vi "SO2 43i Serial Data Recording & DECADEv4.4.vi"() -> ()   [LabVIEW 2014]
uses:
  <vilib>/Instr/_visa.llb/VISA Set IO Buffer Mask.ctl
  <vilib>/Platform/TimedLoop/XDataNode/timing_clust.ctl
  <vilib>/Platform/TimedLoop/XDataNode/nitl_modes.ctl
  <vilib>/Platform/TimedLoop/XDataNode/wakeup.ctl
  C:/Program Files (x86)/National Instruments/LabVIEW 2014/examples/Data Communication/Network Streams/Simple Network Streams/support/Network Stream Command.ctl
  <vilib>/Utility/error.llb/whitespace.ctl
  <vilib>/Instr/_visa.llb/VISA Configure Serial Port (Instr).vi
  <vilib>/Utility/file.llb/Read From Spreadsheet File (string).vi
  <vilib>/Utility/tcp.llb/UDP Multicast Write-Only Open.vi
  <vilib>/platform/TimedLoop/XDataNode/XDataNode.xnode
  <vilib>/Platform/TimedLoop/XDataNode/XDNodeRunTimeDep.lvlib
  <vilib>/ptbypt/NI_PtbyPt.lvlib
panel:
  out "ASCII_file_out":string
  out "local\ndummy":bool
  out "cal gas cylinder conc":dbl=500.0 format="%.4g"
  out "calcon save to file":bool
  out "ev8 zero interval":i32=600
  out "Auto Zeroing":bool
  out "Simulate MOCCA Conc":dbl
  out "MOCCA window delay time (sec)":i32=30
  out "MOCCA SO2 Limit":i32=800
  out "SO2 Inflight MOCCA Alarm\n(default = OFF)":bool
  out "ev8 user set time":i32=60
  out "Mean Cal Offset":dbl
  out "Mean Cal\n(default = ON)":bool=TRUE
  out "Default file name":string
  out "Stop File Write":bool
  out "error out 4":errorcluster
  out "V6":bool
  out "V8":bool
  out "V9":bool
  out "error out 2":errorcluster
  in  "MFC_2 SLPM set value":dbl
  out "Value Read 2":string
  out "status 2":bool
  out "MFC 2":dbl[](array[numeric])
  in  "VISA resource name 3":refnum<visa-resource-name>="ASRL4::INSTR"
  in  "timeout (10sec) 3":u32=3000
  out "error out 3":errorcluster
  in  "MFC_3 SLPM set value":dbl=2.0
  out "Value Read 3":string
  out "status":bool
  out "MFC 3":dbl[](array[numeric])
  in  "VISA resource name 2":refnum<visa-resource-name>="ASRL5::INSTR"
  in  "timeout (10sec) 2":u32=3000
  out "Data Array UDP":string[](array[string])
  out "Slope":dbl=1.1
  out "Zero":dbl
  out "Simulate TWA Conc":dbl
  out "8hr_TWA_limit":i32=490
  out "10mins_STEL_limit":i32=800
  out "Simulate STEL Conc":dbl
  out "Simulate\nconc":bool
  out "q_size 2":i32
  out "8hr_so2_avg 2":dbl=1.0
  out "10min_so2_avg":dbl=1.0
  out "q_size":i32
  in  "Clear Display\nErrors":bool
  out "Data Processing":bool
  out "Serial Visa Error":errorcluster
  out "SEPTIC TCP Error Out":errorcluster
  out "TCP packet\nSend to SEPTIC":bool
  out "UDP Time Stamp Offset":i32=1
  out "Data Array TCP":string[](array[string])
  out "UDP packet \nstatus":bool
  out "UDP_Out_Error":errorcluster
  out "FISH TCP Error Out":errorcluster
  out "TCP packet\nSend to FISH":bool
  out "TCP Binary Packet":string
  out "Scan from String Error Counter\nfrom process loop":i32
  out "Read Error Counter\nfrom process loop":i32
  in  "milliseconds to wait":u32=330
  in  "ID":string="µ"
  in  "VISA resource name":refnum<visa-resource-name>="ASRL6::INSTR"
  out "Data In Array":string[](array[string])
  out "UDP_ASCII_Out":string
  out "UDP_Pack_num":u32
  out "Flight Number":string
  in  "dummy":string="00"
  out "Data String":string
  out "Internal packet":string[](array[string])
  out "RAW DATA":string
  in  "stop":bool
  out "Time taken history":u32(graph)
  out "Max Acq Time diff":u32
  out "Acq Time":u32
  out "Number of Send & Read Error\nfrom Acquire Loop":i32
  out "Command In":string
  # "SO2_conc"
  # "PMT_Volt"
  # "Lamp_Volt"
  # "Lamp_Intensity_Hz"
  # "Internal_Temp_degC"
  # "Reaction_Chamber_Temp_degC"
  # "Reaction_Chamber_Press_mmHg"
  # "Sample_Flow_litre_per_minute"
  # "Flag"
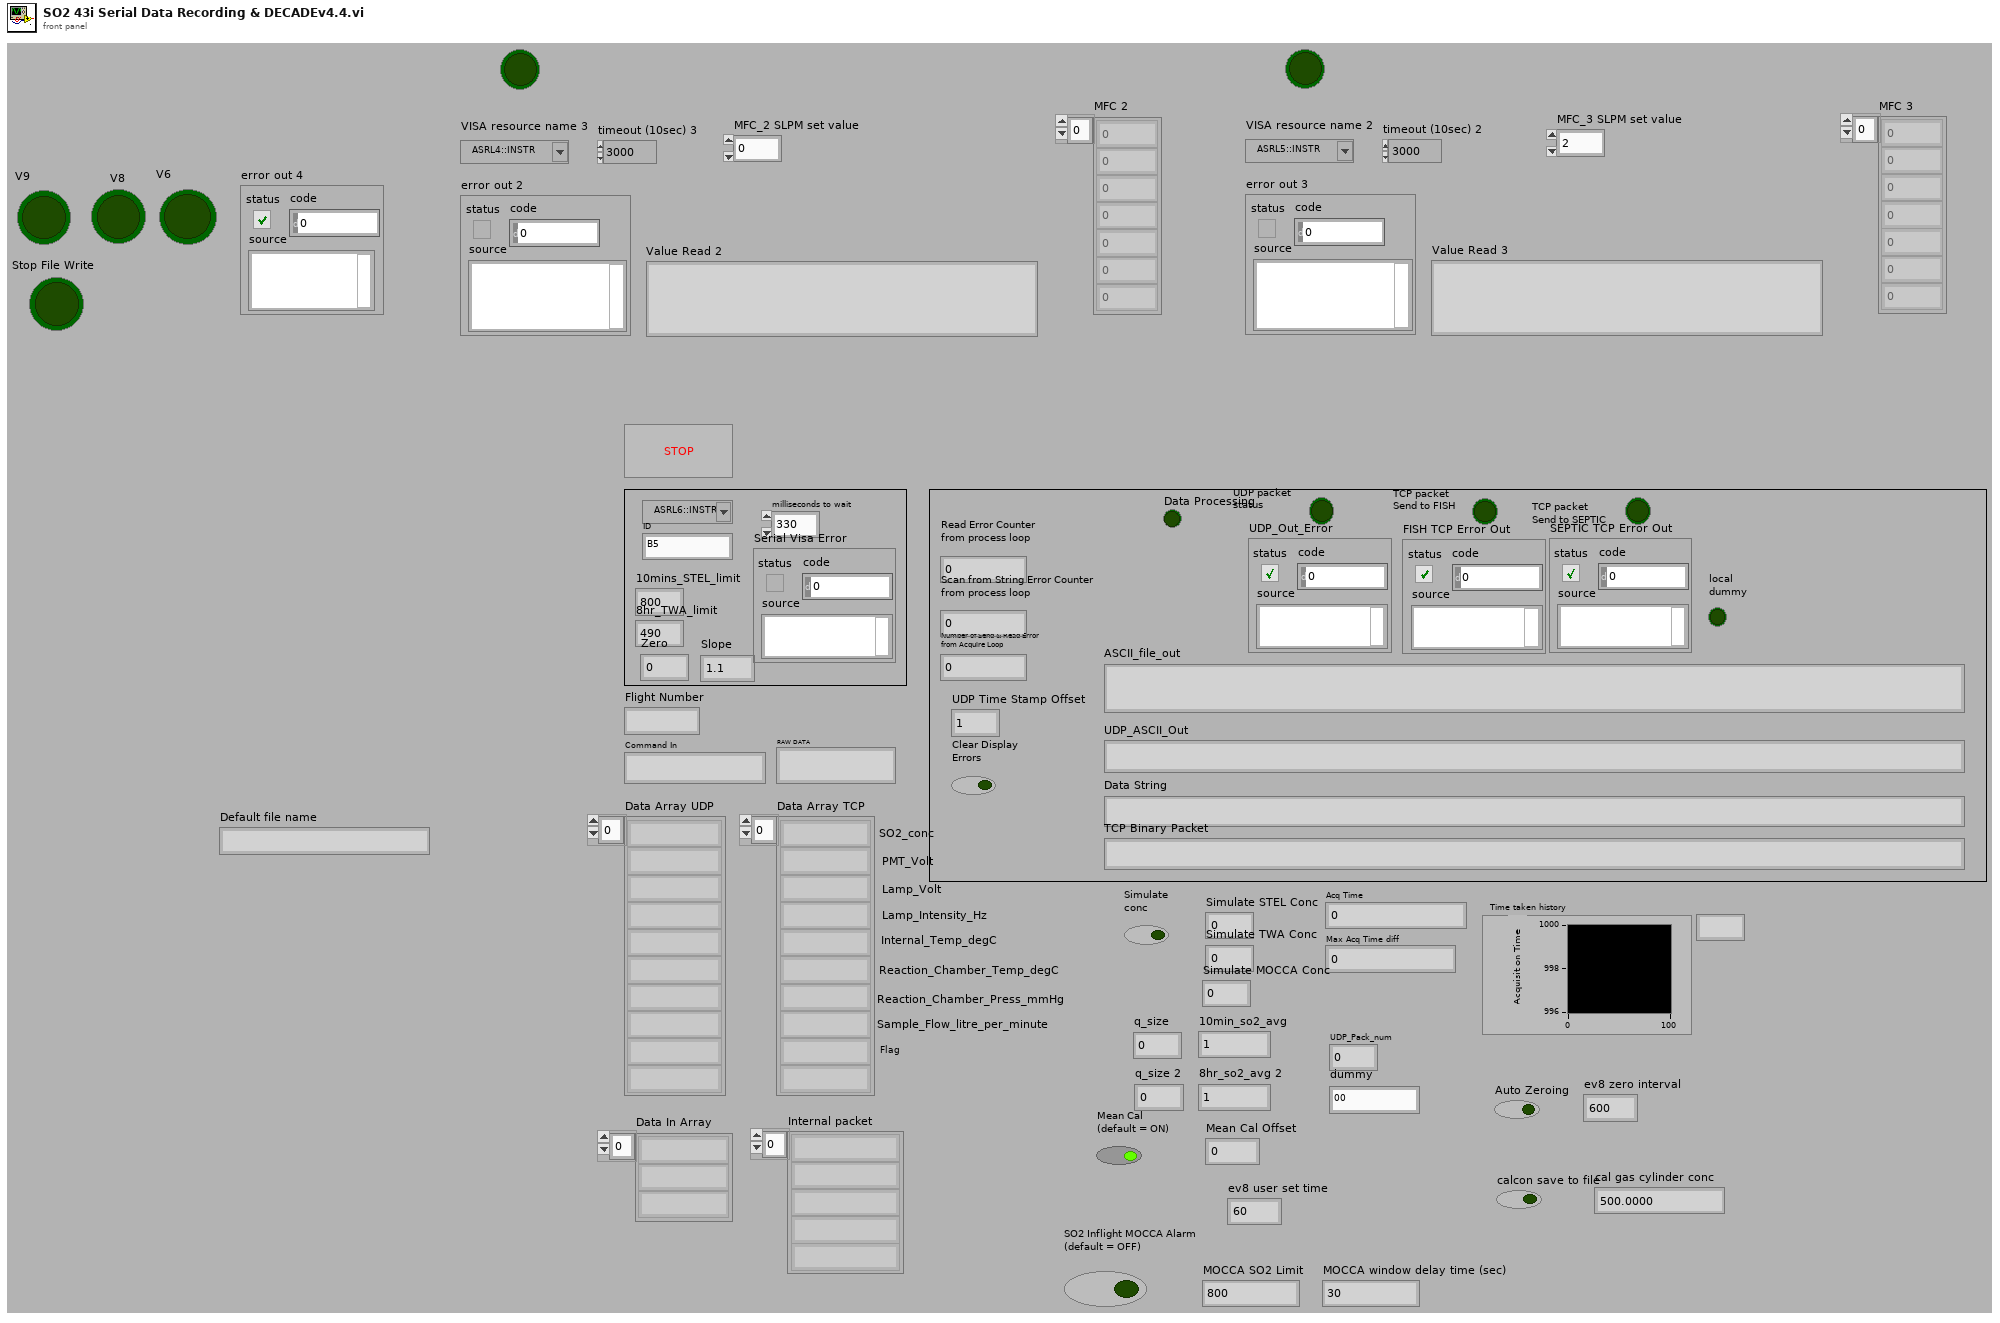
[diagram p1: front panel]
types:
  T1 = typedef "VISA Set IO Buffer Mask.ctl" = u16
  T2 = enum16{"open", "replace", "create", "open or create", "replace or create", "replace or create with confirmation"}
  T3 = typedef "Network Stream Command.ctl" = cluster{"Message":string, "Message Data":variant}
  T4 = typedef "XDNodeRunTimeDep.lvlib/timing_clust.ctl" = cluster{"Expected End [f-1]":u64, "Actual End [f-1]":u64, "Finished Late? [f-1]":bool, "Expected End [i-1]":u64, "Actual End [i-1]":u64, "Finished Late? [i-1]":bool, "Expected Start [i]":u64, "Actual Start [i]":u64, "Expected Start [f]":u64, "Actual Start [f]":u64, "Source Name":string, "Structure Name":string, "Period":i64, "Deadline":i64, "Offset":i64, "Start":i64, "Priority":i32, "Timeout":i32, "Mode":T5, "Wakeup Reason":T6, "Error":errorcluster, "Source Type":string, "Secondary Source Type":string, "Global End Time":u64, "Global Start Time":u64, "Frame Duration":u64, "Iteration Duration":u64, "Assigned CPU":i32, "I/O Scan Engine Mode":u32}
  T5 = typedef "XDNodeRunTimeDep.lvlib/nitl_modes.ctl" = enum32{"No Change", "Process missed periods, maintain original phase", "Discard missed periods, maintain original phase", "Process missed periods, ignore original phase", "Discard missed periods, ignore original phase"}
  T6 = typedef "XDNodeRunTimeDep.lvlib/wakeup.ctl" = enum32{"Normal", "Aborted", "Asynchronous wakeup", "Timing source error", "Timed loop error", "Timeout"}
  T7 = typedef "whitespace.ctl" = u16
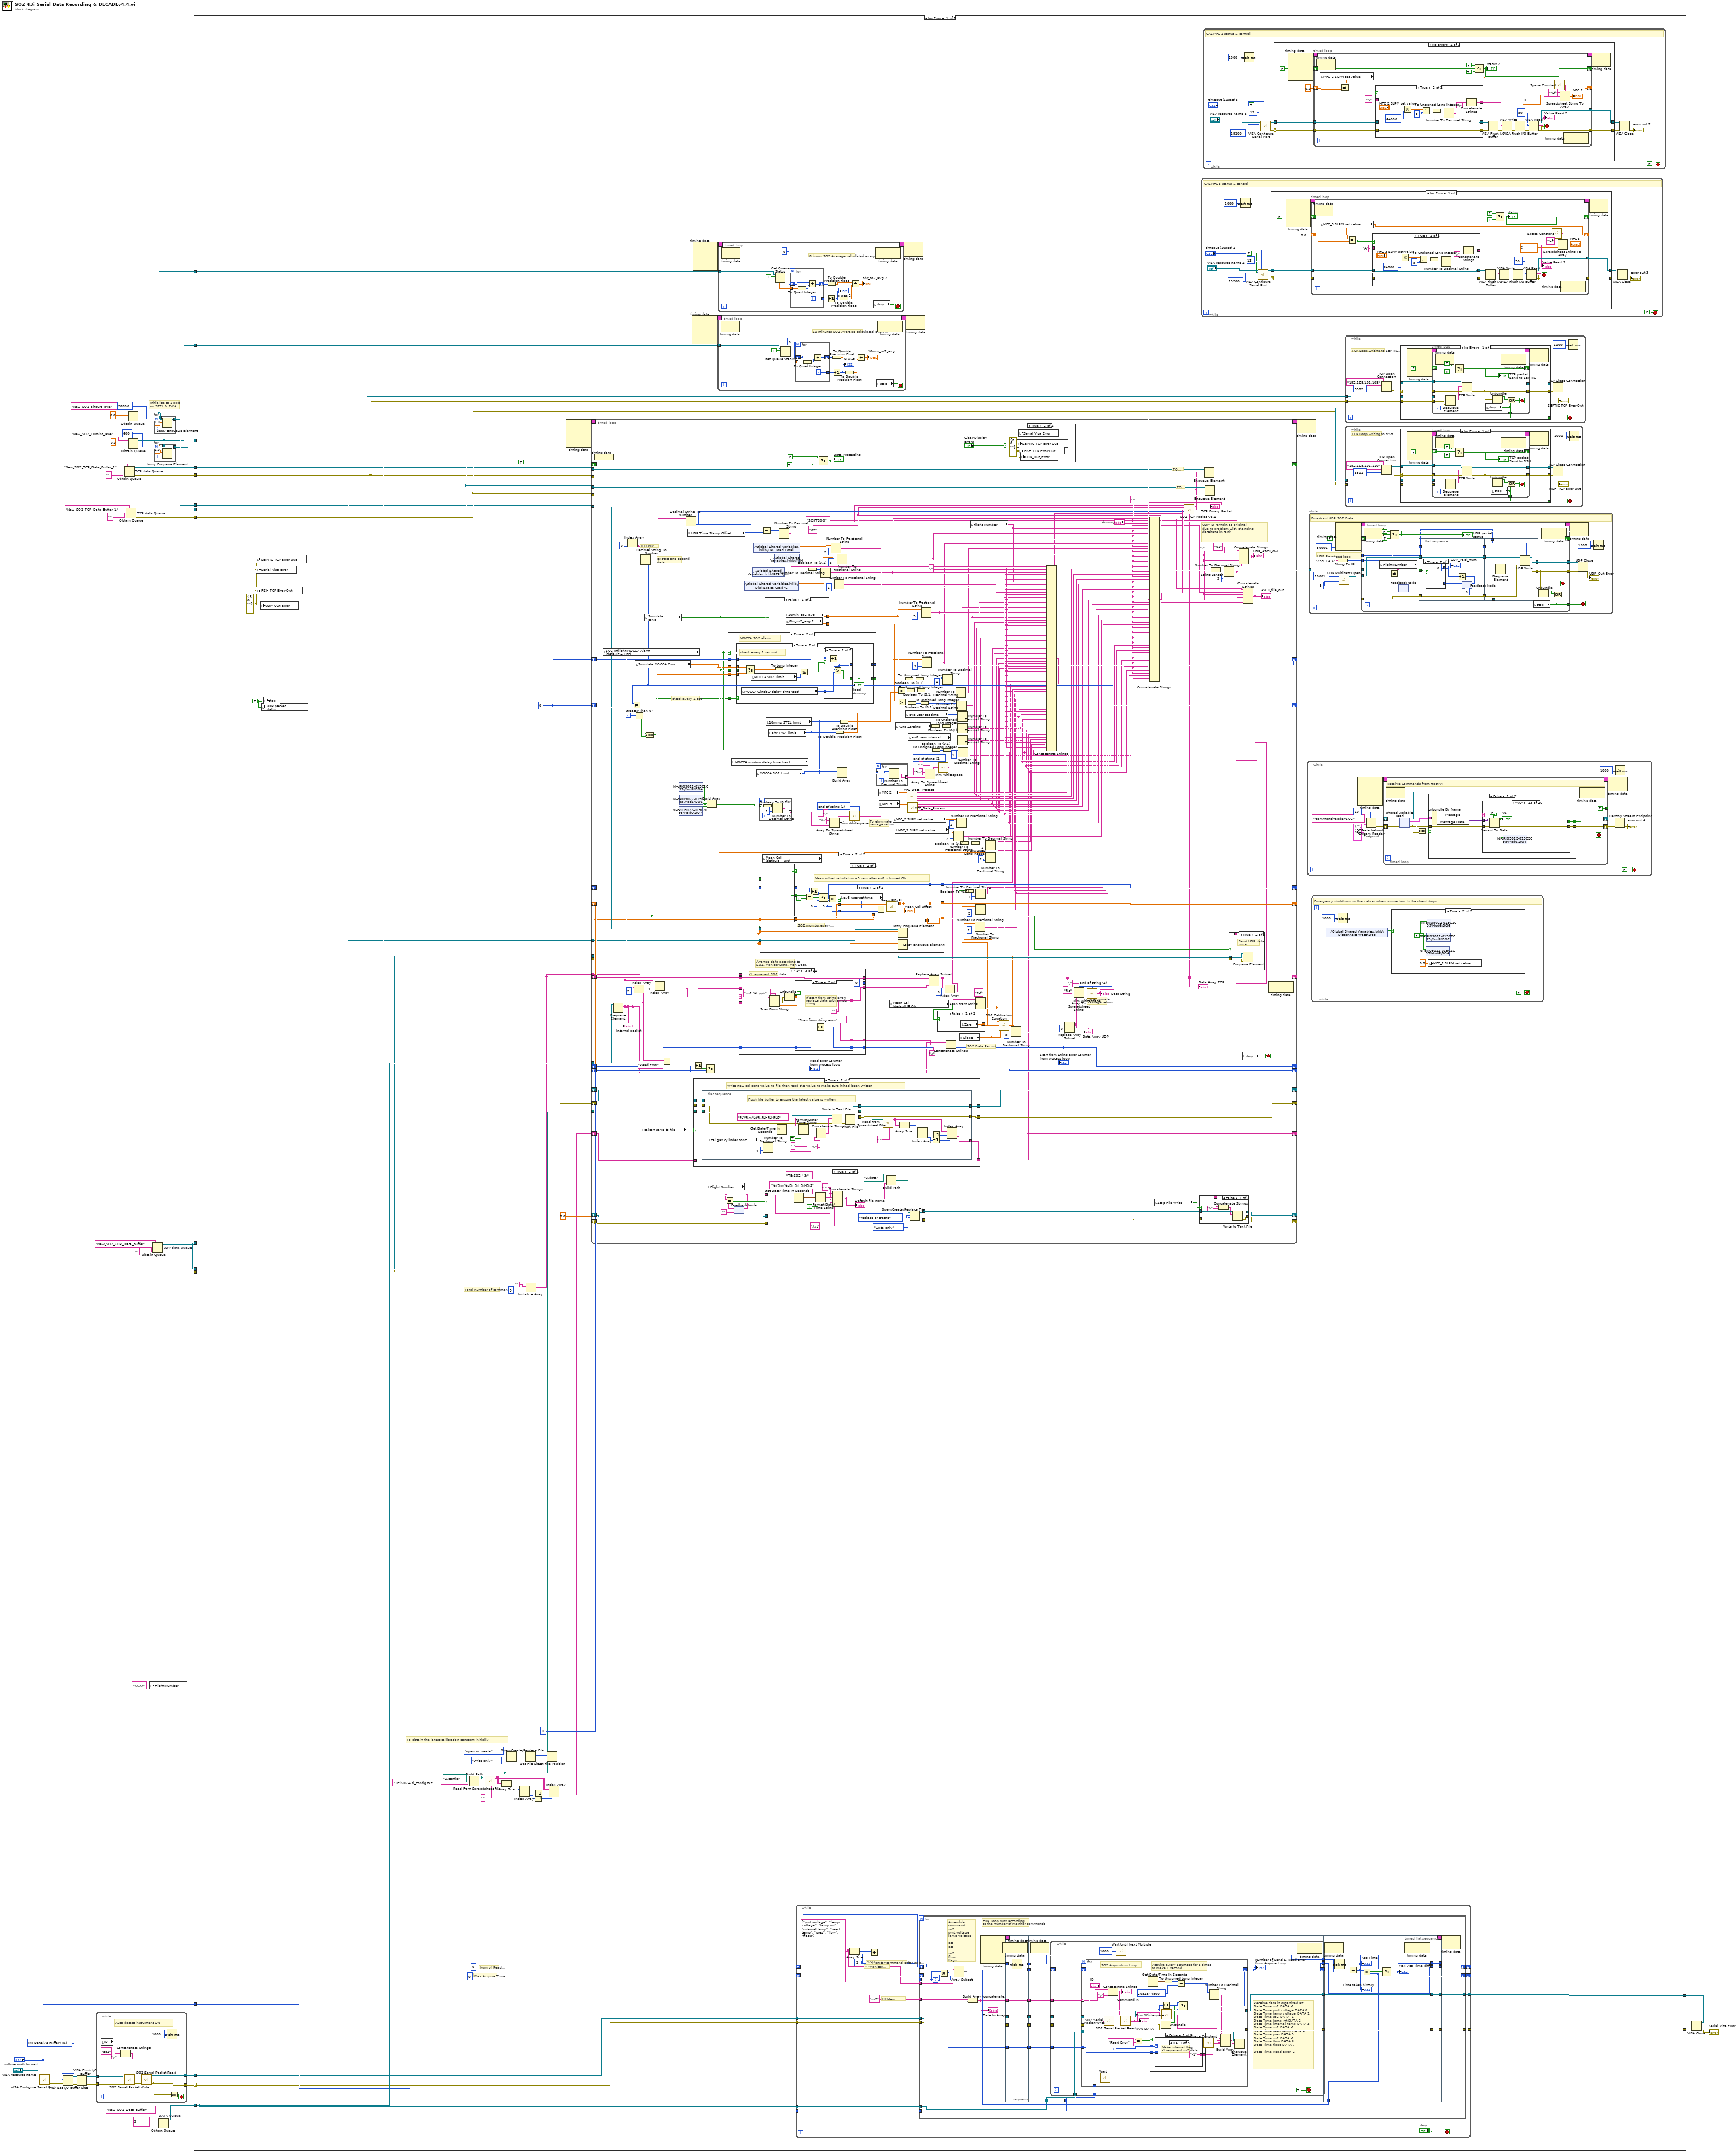
[diagram p0: block diagram]
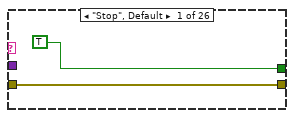
[diagram p3: hidden frame]
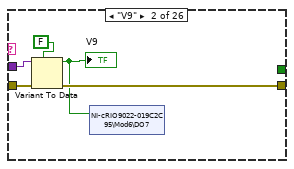
[diagram p4: hidden frame]
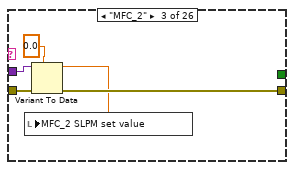
[diagram p5: hidden frame]
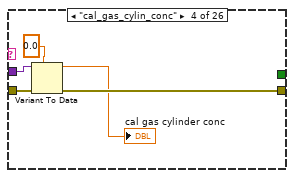
[diagram p6: hidden frame]
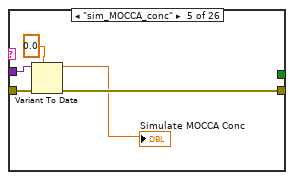
[diagram p7: hidden frame]
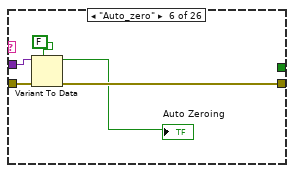
[diagram p8: hidden frame]
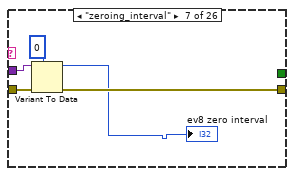
[diagram p9: hidden frame]
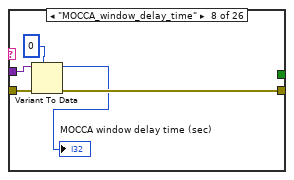
[diagram p10: hidden frame]
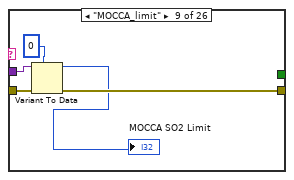
[diagram p11: hidden frame]
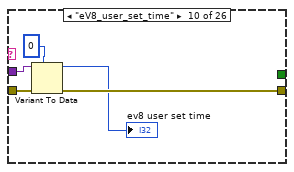
[diagram p12: hidden frame]
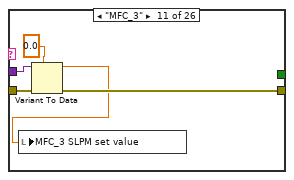
[diagram p13: hidden frame]
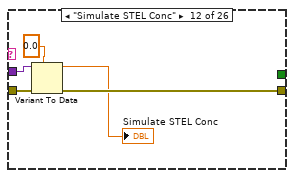
[diagram p14: hidden frame]
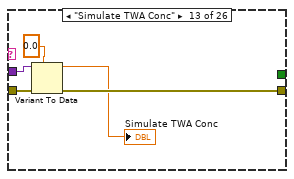
[diagram p15: hidden frame]
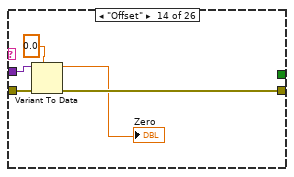
[diagram p16: hidden frame]
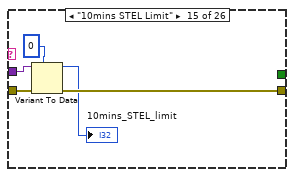
[diagram p17: hidden frame]
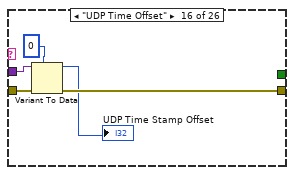
[diagram p18: hidden frame]
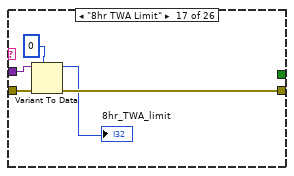
[diagram p19: hidden frame]
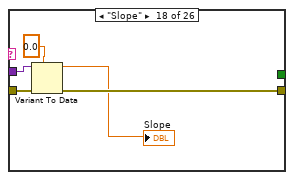
[diagram p20: hidden frame]
diagram:
  w9 = T1 16 items=["I/O Receive Buffer"=16, "I/O Transmit Buffer"=32, "I/O Receive and Transmit Buffer"=48] ("Mask")
  w16 = 28800 ("max queue size (-1, unlimited)")
  w13 = 600 ("max queue size (-1, unlimited)")
  # "Initialise to 1 ppb\non STEL & TWA"
  n1 = call-poly "VISA Configure Serial Port"("VISA resource name"="VISA resource name", "timeout (10sec)"="milliseconds to wait") -> ("VISA resource name out"=w8:refnum<visa-resource-name>, "error out"=w7:errorcluster)  [unwired: 12 in]
  n2 = VISA Set I/O Buffer Size(VISA resource name=w8, mask (16)=w9, error in (no error)=w7) -> (VISA resource name out=w2:refnum<visa-resource-name>, error out=w10:errorcluster)  [unwired: 1 in]
  n3 = VISA Flush I/O Buffer(VISA resource name=w2, error in (no error)=w10) -> (VISA resource name out=w6:refnum<visa-resource-name>, error out=w5:errorcluster)  [unwired: 1 in]
  n4 = while {
    tunnel: w6 -> [w45]
    tunnel: w5 -> [w44]
    tunnel: [w43] -> w4
    tunnel: [w42] -> w3
    stop <- w41 stop-if-true
    # "Auto detect instrument ON"
    n5 = local read "ID"() -> (w46:string)
    n6 = Concatenate Strings(w46, "so2" ("string"), "\r") -> (w49:string)
    n7 = call "SO2 Serial Packet Write.vi"("VISA resource name In"=w45, "Data in"=w49, "error in (no error)"=w44) -> ("VISA resource name Out"=w51:refnum<visa-resource-name>, "error out"=w50:errorcluster)  [unwired: 11 in]
    n8 = call "SO2 Serial Packet Read.vi"("VISA resource In"=w51, "error in"=w50) -> ("VISA resource Out"=w42:refnum<visa-resource-name>, "error out"=w43:errorcluster)  [unwired: 11 in, 1 out]
    n9 = Wait (ms)(milliseconds to wait=u32 1000) -> ()  [unwired: 1 out]
    n10 = Not(x=w43) -> (.not. x?=w41:bool)
  }
  n11 = Obtain Queue "TCP data Queue"(name (unnamed)="New_SO2_TCP_Data_Buffer_2", element data type="") -> (queue out=w23:refnum<queue>, error out=w22:errorcluster)  [unwired: 3 in, 1 out]
  n12 = Obtain Queue "TCP data Queue"(name (unnamed)="New_SO2_TCP_Data_Buffer_1", element data type="") -> (queue out=w31:refnum<queue>, error out=w30:errorcluster)  [unwired: 3 in, 1 out]
  n13 = Obtain Queue(max queue size (-1, unlimited)=w16, name (unnamed)="New_SO2_8hours_ave", element data type=0.0 ("index")) -> (queue out=w15:refnum<queue>)  [unwired: 2 in, 2 out]
  n14 = Obtain Queue(max queue size (-1, unlimited)=w13, name (unnamed)="New_SO2_10mins_ave", element data type=0.0 ("index")) -> (queue out=w12:refnum<queue>)  [unwired: 2 in, 2 out]
  n15 = local write "Flight Number"("XXXX" ("Flight Number")) -> ()
  n16 = Obtain Queue "UDP data Queue"(name (unnamed)="New_SO2_UDP_Data_Buffer", element data type="") -> (queue out=w26:refnum<queue>, error out=w27:errorcluster)  [unwired: 3 in, 1 out]
  n17 = for {
    N: w16 -> [_]
    tunnel: w15 -> [w55]
    tunnel: [w54] -> w14
    n18 = Lossy Enqueue Element(queue=w55, element=1.0) -> (queue out=w54:refnum<queue>)  [unwired: 1 in, 3 out]
  }
  n19 = for {
    N: w13 -> [_]
    tunnel: [w58] -> w11
    tunnel: w12 -> [w56]
    n20 = Lossy Enqueue Element(queue=w56, element=1.0) -> (queue out=w58:refnum<queue>)  [unwired: 1 in, 3 out]
  }
  n21 = Obtain Queue "DATA Queue"(name (unnamed)="New_SO2_Data_Buffer", element data type=string[] []) -> (queue out=w38:refnum<queue>)  [unwired: 3 in, 2 out]
  n22 = case shown="No Error" w4 {
    selector: w4 -> [w81 w1298]
    tunnel: [w112 w1298] -> w35
    tunnel: [w111 w1297] -> w36
    tunnel: w38 -> [w108 _]
    tunnel: w3 -> [w82 w1297]
    tunnel: w31 -> [w100 _]
    tunnel: w30 -> [w99 _]
    tunnel: w26 -> [w98 _]
    tunnel: w27 -> [w97 _]
    tunnel: w26 -> [w96 _]
    tunnel: w23 -> [w95 _]
    tunnel: w22 -> [w94 _]
    tunnel: "milliseconds to wait" -> [w93 _]
    tunnel: w12 -> [w90 _]
    tunnel: w15 -> [w89 _]
    tunnel: w11 -> [w88 _]
    tunnel: w14 -> [w87 _]
    frame No Error {
      w79 = 0
      w91 = errorcluster {"status"=FALSE, "code"=0, "source"=""} ("UDP Error Out")
      w102 = 0
      w101 = FALSE ("stop")
      # "To obtain the latest calibration constant initially"
      # "Max Acquire Time Diff"
      # "Num of Read Error"
      # "Total number of commands"
      n23 = local write "SEPTIC TCP Error Out"(w91) -> ()
      n24 = local write "Serial Visa Error"(w91) -> ()
      n25 = local write "FISH TCP Error Out"(w91) -> ()
      n26 = local write "UDP_Out_Error"(w91) -> ()
      n27 = local write "UDP packet \nstatus"(w101) -> ()
      n28 = local write "stop"(w101) -> ()
      n29 = Build Path(base path=path "u:/config", name or relative path="TEiSO2-43i_config.txt" ("string")) -> (appended path=w61:path)
      n30 = call-poly <vilib>:"Read From Spreadsheet File.vi"("delimiter (\\t)"="," ("delimiter (\\t)"), "file path (dialog if empty)"=w61) -> ("all rows"=w70:string[][])  [unwired: 5 in, 4 out]
      n31 = Array Size(array=w70) -> (size(s)=w71:i32[])
      n32 = Open/Create/Replace File(file path (use dialog)=w61, operation (0:open)=T2."open or create", access (0:read/write)=enum16{"read/write", "read-only", "write-only"}."write-only") -> (refnum out=w63:refnum<file>, error out=w64:errorcluster)  [unwired: 3 in, 1 out]
      n33 = Index Array(array=w71) -> (element #1=w75:i32, element #2=w73:i32)  [unwired: 2 in]
      n34 = Get File Size(file=w63, error in=w64) -> (refnum out=w65:refnum<file>, size (in bytes)=w67:i64, 0:w66:errorcluster)
      n35 = Initialize Array("", 9) -> (w103:string[])
      n36 = Decrement(x=w73) -> (x-1=w72:i32)
      n37 = Decrement(x=w75) -> (x-1=w74:i32)
      n38 = Set File Position(offset (in bytes) (0)=w67, refnum=w65, error in=w66) -> (refnum out=w60:refnum<file>, error out=w59:errorcluster)  [unwired: 1 in]
      n39 = Index Array(array=w70, index (row)=w74, index (col)=w72) -> (element=w69:string)
      n40 = node-c288() -> (w110:T4)  [unwired: 4 in]
      n41 = timed-loop {
        timing: w110 -> [_]
        timing-out: [_] -> w109
        tunnel: w108 -> [w947]
        shift-right: [w745] -> _
        shift-left: w103 -> [w940]
        shift-right: [w931] -> _
        shift-left: w102 -> [w928]
        tunnel: w103 -> [w930]
        shift-right: [w926] -> _
        shift-left: w102 -> [w927]
        tunnel: w100 -> [w924]
        tunnel: w99 -> [w923]
        tunnel: w98 -> [w922]
        tunnel: w97 -> [w921]
        shift-right: [w913] -> _
        shift-left: w79 -> [w916]
        tunnel: w95 -> [w912]
        tunnel: w94 -> [w911]
        shift-right: [w904] -> _
        shift-left: FALSE -> [w907]
        tunnel: w88 -> [w901]
        tunnel: w87 -> [w900]
        shift-right: [w870] -> _
        shift-left: _ -> [w872]
        shift-right: [w869] -> _
        shift-left: _ -> [w871]
        shift-right: [w840] -> _
        shift-left: w79 -> [w842]
        shift-right: [w838] -> _
        shift-left: 0.0 -> [w839]
        shift-right: [w828] -> _
        shift-left: w79 -> [w829]
        tunnel: w61 -> [w805]
        shift-right: [w759] -> _
        shift-left: w69 -> [w804]
        shift-right: [w795] -> _
        shift-left: w60 -> [w796]
        shift-right: [w793] -> _
        shift-left: w59 -> [w794]
        i -> [w914]
        stop <- w945 stop-if-true
        w756 = ","
        (unwired) i16 1 ("width (-)")
        (unwired) T7 2 items=["both", "start of string", "end of string"] ("location (both)")
        w848 = T7 2 items=["both", "start of string", "end of string"] ("location (both)")
        w936 = T7 2 items=["both", "start of string", "end of string"] ("location (both)")
        w798 = ","
        w749 = "02"
        w750 = ","
        w748 = "$CHTSOO"
        # "UDP ID remain as original\ndue to problem with changing\ndatabase in tank"
        # "check every 1 sec"
        # "To eliminate\ncarriage return"
        # "TO SEPTIC"
        # "TO FISH"
        # "Extract one second data\nfor UDP sending"
        # "Arrange data according to\nSO2, Monitor Data, Mon Data,"
        # "To eliminate\ncarriage return"
        # ">>UNIX TIME>>"
        # "SO2 Data Record"
        n42 = node-c288() -> ()  [unwired: 1 in]
        n43 = local read "SO2 Inflight MOCCA Alarm\n(default = OFF)"() -> (w791:bool)
        n44 = Dequeue Element(queue=w947) -> (element=w919:string[])  [unwired: 2 in, 3 out]
        "Internal packet" <- w919
        n45 = Index Array(array=w919, index=0) -> (element=w918:string)
        n46 = Index Array(array=w919, index=2) -> (element=w934:string)
        n47 = Greater Than 0?(x=w914) -> (x > 0?=w917:bool)
        n48 = local read "Simulate MOCCA Conc"() -> (w799:dbl)
        n49 = Decimal String To Number(string=w918) -> (number=w913:i32)  [unwired: 2 in, 1 out]
        n50 = Not Equal?(x=w913, y=w916) -> (x != y?=w915:bool)
        n51 = local read "calcon save to file"() -> (w792:bool)
        n52 = local read "Simulate\nconc"() -> (w801:bool)
        n53 = Compound Arithmetic op=AND(w915, w917) -> (w790:bool)
        n54 = Index Array(array=w919, index=4) -> (element=w903:string)
        n55 = Equal?(x=w934, y="Read Error") -> (x = y?=w932:bool)
        n56 = shared-variable "NI-cRIO9022-019C2C95\\Mod6\\DO7"() -> (w856:bool)  [unwired: 1 in, 1 out]
        n57 = shared-variable "NI-cRIO9022-019C2C95\\Mod6\\DO4"() -> (w857:bool)  [unwired: 1 in, 1 out]
        n58 = shared-variable "NI-cRIO9022-019C2C95\\Mod6\\DO6"() -> (w843:bool)  [unwired: 1 in, 1 out]
        n59 = Decimal String To Number(string=w918) -> (number=w753:i32)  [unwired: 2 in, 1 out]
        n60 = local read "UDP Time Stamp Offset"() -> (w847:i32)
        n61 = Increment(x=w928) -> (x+1=w929:i32)
        n62 = case shown="True" w792 {
          tunnel: w805 -> [_ w959]
          tunnel: [w948 w957] -> w793
          tunnel: w804 -> [w950 _]
          tunnel: [w950 w956] -> w759
          tunnel: w796 -> [w949 w954]
          tunnel: [w949 w952] -> w795
          tunnel: w794 -> [w948 w951]
          frame False {
          }
          frame True {
            # "Write new cal conc value to file then read the value to make sure it had been written"
            n63 = flat-sequence {
              tunnel: w959 -> [w967]
              tunnel: [w962] -> w958
              tunnel: [w967] -> w955
              tunnel: w954 -> [w966]
              tunnel: [w961] -> w953
              tunnel: w951 -> [w965]
              tunnel: w958 -> [w980]
              tunnel: [w980] -> w957
              tunnel: [w979] -> w956
              tunnel: w955 -> [w978]
              tunnel: w953 -> [w977]
              tunnel: [w977] -> w952
              frame #0 {
                # "Flush file buffer to ensure the latest value is written"
                n64 = local read "cal gas cylinder conc"() -> (w960:dbl)
                n65 = Number To Fractional String(number=w960, precision (6)=i16 4) -> (F-format string=w968:string)  [unwired: 2 in]
                n66 = Get Date/Time In Seconds() -> (seconds since 1Jan1904=w975:timestamp)
                n67 = Format Date/Time String(time format string (%c)="%Y%m%d%,%H%M%S", seconds (now)=w975, UTC format=TRUE) -> (date/time string=w972:string)
                n68 = Concatenate Strings(w972, "," ("string"), w968, "\r") -> (w970:string)
                n69 = Write to Text File(file (use dialog)=w966, text=w970, error in=w965) -> (refnum out=w963:refnum<file>, error out=w964:errorcluster)  [unwired: 1 in, 1 out]
                n70 = Flush File(refnum=w963, error in=w964) -> (refnum out=w961:refnum<file>, error out=w962:errorcluster)
              }
              frame #1 {
                n71 = call-poly <vilib>:"Read From Spreadsheet File.vi"("delimiter (\\t)"="," ("delimiter (\\t)"), "file path (dialog if empty)"=w978) -> ("all rows"=w981:string[][])  [unwired: 5 in, 4 out]
                n72 = Array Size(array=w981) -> (size(s)=w982:i32[])
                n73 = Index Array(array=w982) -> (element #1=w986:i32, element #2=w984:i32)  [unwired: 2 in]
                n74 = Decrement(x=w984) -> (x-1=w983:i32)
                n75 = Decrement(x=w986) -> (x-1=w985:i32)
                n76 = Index Array(array=w981, index (row)=w985, index (col)=w983) -> (element=w979:string)
              }
            }
          }
        }
        n77 = Select(t=w929, s=w932, f=w928) -> (s? t:f=w931:i32)
        "Read Error Counter\nfrom process loop" <- w931
        n78 = Build Array(w857, w843, w856) -> (w861:bool[])
        n79 = local read "Flight Number"() -> (w873:string)
        n80 = local read "MOCCA window delay time (sec)"() -> (w810:i32)
        n81 = feedback #1("" ("Flight Number")) -> (w878:string)
        n82 = Not Equal?(x=w873, y=w878) -> (x != y?=w876:bool)
        n83 = feedback-in #1(w873) -> ()
        n84 = case shown="\"-1\"" w903 {
          tunnel: w903 -> [w1096 _ _ w1132 w1153 w1174 w1196 w1218 w1240 w1262 w1284]
          tunnel: w940 -> [w1097 _ w1111 w1133 w1154 w1175 w1197 w1219 w1241 w1263 w1285]
          tunnel: w934 -> [_ _ w1108 w1128 w1149 w1171 w1193 w1215 w1237 w1259 w1281]
          tunnel: [w1097 w1100 w1111 w1133 w1154 w1175 w1197 w1219 w1241 w1263 w1285] -> w887
          tunnel: [w1094 _ 0 ("index") w1130 w1151 w1172 w1194 w1216 w1238 w1260 w1282] -> w886
          tunnel: [_ _ w1107 w1127 w1148 w1170 w1192 w1214 w1236 w1258 w1276] -> w939
          tunnel: w930 -> [_ w1100 _ _ _ _ _ _ _ _ _]
          tunnel: w927 -> [w1092 w1099 w1104 w1124 w1145 w1165 w1188 w1209 w1232 w1253 w1275]
          tunnel: [w1092 w1099 w1103 w1123 w1144 w1164 w1187 w1208 w1231 w1252 w1274] -> w926
          tunnel: ["Internal False Flag Detected" "" w1102 w1122 w1143 w1163 w1186 w1207 w1230 w1251 w1273] -> w925
          frame "False", Default {
            n85 = Decimal String To Number(string=w1096) -> (number=w1093:i32)  [unwired: 2 in, 1 out]
            n86 = Add(x=w1093, y=1) -> (x+y=w1094:i32)
          }
          frame "-2" {
            # "Read Error Detected\nMake all data as a space"
          }
          frame "-1" {
            # "-1 represent SO2 data"
            n87 = Scan From String(format string="so2 %f ppb", input string=w1108) -> (error out=w1106:errorcluster, output 1=w1101:dbl)  [unwired: 3 in, 2 out]
            n88 = Unbundle(w1106) -> ("status"=w1105:bool)  [unwired: 2 out]
            n89 = case shown="True" w1105 {
              tunnel: w1101 -> [w1112 _]
              tunnel: [w1116 ""] -> w1107
              tunnel: w1104 -> [w1115 w1120]
              tunnel: [w1115 w1119] -> w1103
              tunnel: ["" "Scan from string error"] -> w1102
              frame False {
                # "Extract the concentration\nvalue & fixed format"
                n90 = Number To Fractional String(number=w1112, precision (6)=i16 5) -> (F-format string=w1116:string)  [unwired: 2 in]
              }
              frame True {
                # "If scan from string error,\nreplace data with empty\nstring"
                n91 = Increment(x=w1120) -> (x+1=w1119:i32)
              }
            }
          }
          frame "0" {
            # "0 represents pmt voltage -0510 volts"
            n92 = Scan From String(format string="pmt voltage %d", input string=w1128) -> (error out=w1126:errorcluster, output 1=w1121:i32)  [unwired: 3 in, 2 out]
            n93 = Decimal String To Number(string=w1132) -> (number=w1131:i32)  [unwired: 2 in, 1 out]
            n94 = Unbundle(w1126) -> ("status"=w1125:bool)  [unwired: 2 out]
            n95 = case shown="False" w1125 {
              tunnel: w1121 -> [w1137 _]
              tunnel: [w1134 w1138] -> w1127
              tunnel: w1124 -> [w1136 w1141]
              tunnel: [w1136 w1140] -> w1123
              tunnel: ["" "Scan from string error"] -> w1122
              tunnel: [w1134 w1138] -> _
              frame False {
                # "Extract the actual value\n& fixed format"
                n96 = Number To Decimal String(number=w1137) -> (decimal integer string=w1134:string)  [unwired: 1 in]
              }
              frame True {
                w1138 = ""
                # "If scan from string error,\nreplace data with empty\nstring"
                n97 = Increment(x=w1141) -> (x+1=w1140:i32)
              }
            }
            n98 = Increment(x=w1131) -> (x+1=w1130:i32)
          }
          frame "1" {
            # "1 represents lamp voltage; lamp voltage 810 volts"
            n99 = Scan From String(format string="lamp voltage %d", input string=w1149) -> (error out=w1147:errorcluster, output 1=w1142:i32)  [unwired: 3 in, 2 out]
            n100 = Decimal String To Number(string=w1153) -> (number=w1152:i32)  [unwired: 2 in, 1 out]
            n101 = Unbundle(w1147) -> ("status"=w1146:bool)  [unwired: 2 out]
            n102 = case shown="True" w1146 {
              tunnel: w1142 -> [w1158 _]
              tunnel: [w1155 w1159] -> w1148
              tunnel: w1145 -> [w1157 w1162]
              tunnel: [w1157 w1161] -> w1144
              tunnel: ["" "Scan from string error"] -> w1143
              tunnel: [w1155 w1159] -> _
              frame False {
                # "Extract the actual value\n& fixed format"
                n103 = Number To Decimal String(number=w1158) -> (decimal integer string=w1155:string)  [unwired: 1 in]
              }
              frame True {
                w1159 = ""
                # "If scan from string error,\nreplace data with empty\nstring"
                n104 = Increment(x=w1162) -> (x+1=w1161:i32)
              }
            }
            n105 = Increment(x=w1152) -> (x+1=w1151:i32)
          }
          frame "2" {
            # "2 represents lamp intensity; lamp int 35867 Hz"
            n106 = Scan From String(format string="lamp int %d", input string=w1171) -> (error out=w1167:errorcluster, output 1=w1168:i32)  [unwired: 3 in, 2 out]
            n107 = Decimal String To Number(string=w1174) -> (number=w1173:i32)  [unwired: 2 in, 1 out]
            n108 = Unbundle(w1167) -> ("status"=w1166:bool)  [unwired: 2 out]
            n109 = case shown="True" w1166 {
              tunnel: [w1176 w1181] -> w1170
              tunnel: w1168 -> [w1180 _]
              tunnel: w1165 -> [w1179 w1184]
              tunnel: [w1179 w1183] -> w1164
              tunnel: ["" "Scan from string error"] -> w1163
              tunnel: [w1176 w1181] -> _
              frame False {
                # "Extract the actual value\n& fixed format"
                n110 = Number To Fractional String(number=w1180, precision (6)=i16 0) -> (F-format string=w1176:string)  [unwired: 2 in]
              }
              frame True {
                w1181 = ""
                # "If scan from string error,\nreplace data with empty\nstring"
                n111 = Increment(x=w1184) -> (x+1=w1183:i32)
              }
            }
            n112 = Increment(x=w1173) -> (x+1=w1172:i32)
          }
          frame "3" {
            # "3 represents internal temp; internal temp 027.2 deg C, actual 027.2"
            n113 = Scan From String(format string="%[^,], %s %f", input string=w1193) -> (error out=w1190:errorcluster, output 3=w1185:dbl)  [unwired: 7 in, 2 out]
            n114 = Decimal String To Number(string=w1196) -> (number=w1195:i32)  [unwired: 2 in, 1 out]
            n115 = Unbundle(w1190) -> ("status"=w1189:bool)  [unwired: 2 out]
            n116 = case shown="True" w1189 {
              tunnel: [w1198 w1203] -> w1192
              tunnel: w1185 -> [w1202 _]
              tunnel: w1188 -> [w1201 w1206]
              tunnel: [w1201 w1205] -> w1187
              tunnel: ["" "Scan from string error"] -> w1186
              tunnel: [w1198 w1203] -> _
              frame False {
                # "Extract the actual value\n& fixed format"
                n117 = Number To Fractional String(number=w1202, precision (6)=i16 1) -> (F-format string=w1198:string)  [unwired: 2 in]
              }
              frame True {
                w1203 = ""
                # "If scan from string error,\nreplace data with empty\nstring"
                n118 = Increment(x=w1206) -> (x+1=w1205:i32)
              }
            }
            n119 = Increment(x=w1195) -> (x+1=w1194:i32)
          }
          frame "4" {
            # "4 represents react temp; react temp 045.2 deg C"
            n120 = Scan From String(format string="react temp %f deg C", input string=w1215) -> (error out=w1211:errorcluster, output 1=w1212:dbl)  [unwired: 3 in, 2 out]
            n121 = Decimal String To Number(string=w1218) -> (number=w1217:i32)  [unwired: 2 in, 1 out]
            n122 = Unbundle(w1211) -> ("status"=w1210:bool)  [unwired: 2 out]
            n123 = case shown="False" w1210 {
              tunnel: [w1220 w1225] -> w1214
              tunnel: w1212 -> [w1224 _]
              tunnel: w1209 -> [w1223 w1228]
              tunnel: [w1223 w1227] -> w1208
              tunnel: ["" "Scan from string error"] -> w1207
              tunnel: [w1220 w1225] -> _
              frame False {
                # "Extract the actual value\n& fixed format"
                n124 = Number To Fractional String(number=w1224, precision (6)=i16 1) -> (F-format string=w1220:string)  [unwired: 2 in]
              }
              frame True {
                w1225 = ""
                # "If scan from string error,\nreplace data with empty\nstring"
                n125 = Increment(x=w1228) -> (x+1=w1227:i32)
              }
            }
            n126 = Increment(x=w1217) -> (x+1=w1216:i32)
          }
          frame "5" {
            # "5 represents chamber pressure; pres 760.0 mm Hg, actual 753.4"
            n127 = Scan From String(format string="%[^,], %s %f", input string=w1237) -> (error out=w1234:errorcluster, output 3=w1229:dbl)  [unwired: 7 in, 2 out]
            n128 = Decimal String To Number(string=w1240) -> (number=w1239:i32)  [unwired: 2 in, 1 out]
            n129 = Unbundle(w1234) -> ("status"=w1233:bool)  [unwired: 2 out]
            n130 = case shown="False" w1233 {
              tunnel: [w1242 w1247] -> w1236
              tunnel: w1229 -> [w1246 _]
              tunnel: w1232 -> [w1245 w1250]
              tunnel: [w1245 w1249] -> w1231
              tunnel: ["" "Scan from string error"] -> w1230
              tunnel: [w1242 w1247] -> _
              frame False {
                # "Extract the actual value\n& fixed format"
                n131 = Number To Fractional String(number=w1246, precision (6)=i16 1) -> (F-format string=w1242:string)  [unwired: 2 in]
              }
              frame True {
                w1247 = ""
                # "If scan from string error,\nreplace data with empty\nstring"
                n132 = Increment(x=w1250) -> (x+1=w1249:i32)
              }
            }
            n133 = Increment(x=w1239) -> (x+1=w1238:i32)
          }
          frame "6" {
            # "6 represents flow data; flow 0.503 l/m"
            n134 = Scan From String(format string="flow %f l/m", input string=w1259) -> (error out=w1255:errorcluster, output 1=w1256:dbl)  [unwired: 3 in, 2 out]
            n135 = Decimal String To Number(string=w1262) -> (number=w1261:i32)  [unwired: 2 in, 1 out]
            n136 = Unbundle(w1255) -> ("status"=w1254:bool)  [unwired: 2 out]
            n137 = case shown="True" w1254 {
              tunnel: [w1268 ""] -> w1258
              tunnel: w1256 -> [w1267 _]
              tunnel: w1253 -> [w1266 w1271]
              tunnel: [w1266 w1270] -> w1252
              tunnel: ["" "Scan from string error"] -> w1251
              frame False {
                # "Extract the actual value\n& fixed format"
                n138 = Number To Fractional String(number=w1267, precision (6)=i16 3) -> (F-format string=w1268:string)  [unwired: 2 in]
              }
              frame True {
                # "If scan from string error,\nreplace data with empty\nstring"
                n139 = Increment(x=w1271) -> (x+1=w1270:i32)
              }
            }
            n140 = Increment(x=w1261) -> (x+1=w1260:i32)
          }
          frame "7" {
            # "7 represents flags data; flags 1c100000"
            n141 = Scan From String(format string="flags %s", input string=w1281) -> (error out=w1279:errorcluster, output 1=w1277:string)  [unwired: 3 in, 2 out]
            n142 = Decimal String To Number(string=w1284) -> (number=w1283:i32)  [unwired: 2 in, 1 out]
            n143 = Unbundle(w1279) -> ("status"=w1278:bool)  [unwired: 2 out]
            n144 = case shown="False" w1278 {
              tunnel: w1277 -> [w1288 _]
              tunnel: [w1288 ""] -> w1276
              tunnel: w1275 -> [w1287 w1291]
              tunnel: [w1287 w1290] -> w1274
              tunnel: ["" "Scan from string error"] -> w1273
              frame False {
                # "Extract the actual value\n& fixed format"
              }
              frame True {
                # "If scan from string error,\nreplace data with empty\nstring"
                n145 = Increment(x=w1291) -> (x+1=w1290:i32)
              }
            }
            n146 = Increment(x=w1283) -> (x+1=w1282:i32)
          }
        }
        "Scan from String Error Counter\nfrom process loop" <- w926
        n147 = shared-variable ".\\Global Shared Variables.lvlib\\Disk Space Used %"() -> (w850:dbl)  [unwired: 1 in, 1 out]
        n148 = shared-variable ".\\Global Shared Variables.lvlib\\PTP Sync"() -> (w863:bool)  [unwired: 1 in, 1 out]
        n149 = shared-variable ".\\Global Shared Variables.lvlib\\CPU Load Total"() -> (w867:dbl)  [unwired: 1 in, 1 out]
        n150 = local read "MOCCA SO2 Limit"() -> (w809:i32)
        n151 = for {
          tunnel: w861 -> [w1026] mode=indexing
          tunnel: [w1025] -> w858 mode=indexing
          n152 = Boolean To (0,1)(Boolean=w1026) -> (0, 1=w1027:i16)
          n153 = Number To Decimal String(number=w1027, width (-)=i16 1) -> (decimal integer string=w1025:string)
        }
        n154 = Subtract(x=w753, y=w847) -> (x-y=w909:i32)
        n155 = case shown="False" w801 {
          tunnel: [w1019 w1020] -> w896
          tunnel: [w1018 w1021] -> w894
          frame False {
            n156 = local read "10min_so2_avg"() -> (w1019:dbl)
            n157 = local read "8hr_so2_avg 2"() -> (w1018:dbl)
          }
          frame True {
            # "SO2 STEL & TWA simulate"
            n158 = local read "Simulate STEL Conc"() -> (w1020:dbl)
            n159 = local read "Simulate TWA Conc"() -> (w1021:dbl)
          }
        }
        n160 = case shown="True" w876 {
          tunnel: [w1029 w1032] -> w875
          tunnel: [w1028 w1031] -> w874
          tunnel: w872 -> [w1029 _]
          tunnel: w871 -> [w1028 _]
          tunnel: w873 -> [_ w1030]
          frame False {
          }
          frame True {
            w1039 = "_" ("string")
            n161 = Get Date/Time In Seconds() -> (seconds since 1Jan1904=w1040:timestamp)
            n162 = Format Date/Time String(time format string (%c)="%Y%m%d%_%H%M%S", seconds (now)=w1040, UTC format=TRUE) -> (date/time string=w1043:string)
            n163 = Concatenate Strings("TEiSO2-43i" ("string"), w1039, w1043, w1039, w1030, ".txt" ("string")) -> (w1037:string)
            "Default file name" <- w1037
            n164 = Build Path(base path=path "u:/data", name or relative path=w1037) -> (appended path=w1033:path)
            n165 = Open/Create/Replace File(file path (use dialog)=w1033, operation (0:open)=T2."replace or create", access (0:read/write)=enum16{"read/write", "read-only", "write-only"}."write-only") -> (refnum out=w1032:refnum<file>, error out=w1031:errorcluster)  [unwired: 3 in, 1 out]
          }
        }
        n166 = local read "10mins_STEL_limit"() -> (w808:i32)
        n167 = local read "8hr_TWA_limit"() -> (w807:i32)
        n168 = shared-variable ".\\Global Shared Variables.lvlib\\MFM"() -> (w864:dbl)  [unwired: 1 in, 1 out]
        n169 = Number To Decimal String(number=w909) -> (decimal integer string=w908:string)  [unwired: 1 in]
        n170 = Boolean To (0,1)(Boolean=w863) -> (0, 1=w862:i16)
        n171 = Select(t=FALSE, s=w907, f=TRUE) -> (s? t:f=w904:bool)
        "Data Processing" <- w904
        n172 = Number To Decimal String(number=w862) -> (decimal integer string=w789:string)  [unwired: 1 in]
        n173 = Array To Spreadsheet String(delimiter (Tab)=",", array=w858, 3:"%s" ("format string")) -> (spreadsheet string=w849:string)
        n174 = Number To Fractional String(number=w867, precision (6)=i16 2) -> (F-format string=w846:string)  [unwired: 2 in]
        n175 = Number To Fractional String(number=w850, precision (6)=i16 1) -> (F-format string=w845:string)  [unwired: 2 in]
        n176 = To Double Precision Float(number=w807) -> (double precision float=w897:dbl)
        n177 = Number To Fractional String(number=w864, precision (6)=i16 3) -> (F-format string=w781:string)  [unwired: 2 in]
        n178 = Build Array(w810, w809, w808, w807) -> (w806:i32[])
        n179 = To Double Precision Float(number=w808) -> (double precision float=w898:dbl)
        n180 = call <vilib>:"Trim Whitespace.vi"("string"=w849, "location (both)"=w848) -> ("trimmed string"=w770:string)
        n181 = for {
          tunnel: w806 -> [w988] mode=indexing
          tunnel: [w989] -> w812 mode=indexing
          n182 = Number To Decimal String(number=w988) -> (decimal integer string=w989:string)  [unwired: 1 in]
        }
        n183 = local read "MFC 2"() -> (w880:dbl[])
        n184 = local read "MFC 3"() -> (w879:dbl[])
        n185 = local read "Mean Cal\n(default = ON)"() -> (w834:bool)
        n186 = local read "MFC_2 SLPM set value"() -> (w853:dbl)
        n187 = local read "MFC_3 SLPM set value"() -> (w852:dbl)
        n188 = local read "Auto Zeroing"() -> (w820:bool)
        n189 = Greater?(x=w896, y=w898) -> (0:w891:bool)
        n190 = Greater?(x=w894, y=w897) -> (0:w890:bool)
        n191 = Boolean To (0,1)(Boolean=w891) -> (0, 1=w893:i16)
        n192 = local read "ev8 user set time"() -> (w823:i32)
        n193 = Boolean To (0,1)(Boolean=w890) -> (0, 1=w892:i16)
        n194 = call "MFC_Data_Process.vi"("MFC"=w880) -> ("MFC Absolute Pressure"=w780:string, "MFC Temperature"=w779:string, "MFC Volumetric Flow"=w778:string, "MFC Mass Flow"=w777:string, "MFC Set Point"=w776:string)  [unwired: 10 in]
        n195 = call "MFC_Data_Process.vi"("MFC"=w879) -> ("MFC Absolute Pressure"=w775:string, "MFC Temperature"=w774:string, "MFC Volumetric Flow"=w773:string, "MFC Mass Flow"=w772:string, "MFC Set Point"=w771:string)  [unwired: 10 in]
        n196 = local read "ev8 zero interval"() -> (w819:i32)
        n197 = To Unsigned Long Integer(number=w893) -> (unsigned 32bit integer=w889:u32)
        n198 = To Unsigned Long Integer(number=w892) -> (unsigned 32bit integer=w888:u32)
        n199 = Number To Fractional String(number=w896, precision (6)=i16 5) -> (F-format string=w785:string)  [unwired: 2 in]
        n200 = Number To Fractional String(number=w894, precision (6)=i16 5) -> (F-format string=w784:string)  [unwired: 2 in]
        n201 = Array To Spreadsheet String(delimiter (Tab)=",", array=w812, 3:"%s" ("format string")) -> (spreadsheet string=w811:string)
        n202 = Replace Array Subset(array=w887, new element=w939, index=w886) -> (w745:string[])
        "Data Array TCP" <- w745
        n203 = Boolean To (0,1)(Boolean=w820) -> (0, 1=w822:i16)
        n204 = Boolean To (0,1)(Boolean=w791) -> (0, 1=w818:i16)
        n205 = case shown="False" w834 {
          tunnel: [w1022 w1023] -> w831
          frame False {
            n206 = local read "Zero"() -> (w1022:dbl)
          }
          frame True {
            n207 = local read "Mean Cal Offset"() -> (w1023:dbl)
          }
        }
        n208 = call <vilib>:"Trim Whitespace.vi"("string"=w811) -> ("trimmed string"=w760:string)  [unwired: 1 in]
        n209 = To Unsigned Long Integer(number=w822) -> (unsigned 32bit integer=w821:u32)
        n210 = To Unsigned Long Integer(number=w818) -> (unsigned 32bit integer=w817:u32)
        n211 = Index Array(array=w745, index=0) -> (element=w837:string)
        n212 = Concatenate Strings(w919, w925, "\r") -> ()  [unwired: 1 out]
        n213 = Number To Fractional String(number=w852, precision (6)=i16 2) -> (F-format string=w768:string)  [unwired: 2 in]
        n214 = Number To Decimal String(number=w889) -> (decimal integer string=w783:string)  [unwired: 1 in]
        n215 = Number To Decimal String(number=w888) -> (decimal integer string=w782:string)  [unwired: 1 in]
        n216 = Number To Fractional String(number=w853, precision (6)=i16 2) -> (F-format string=w769:string)  [unwired: 2 in]
        n217 = Number To Decimal String(number=w823) -> (decimal integer string=w764:string)  [unwired: 1 in]
        n218 = Number To Decimal String(number=w821, width (-)=i16 1) -> (decimal integer string=w763:string)
        n219 = Number To Decimal String(number=w819) -> (decimal integer string=w762:string)  [unwired: 1 in]
        n220 = Number To Decimal String(number=w817, width (-)=i16 1) -> (decimal integer string=w761:string)
        n221 = Boolean To (0,1)(Boolean=w801) -> (0, 1=w803:i16)
        n222 = local read "Slope"() -> (w830:dbl)
        n223 = Boolean To (0,1)(Boolean=w834) -> (0, 1=w836:i16)
        n224 = local read "Flight Number"() -> (w787:string)
        n225 = To Unsigned Long Integer(number=w803) -> (unsigned 32bit integer=w802:u32)
        n226 = Number To Fractional String(number=w830, precision (6)=i16 2) -> (F-format string=w765:string)  [unwired: 2 in]
        n227 = Number To Decimal String(number=w836, width (-)=i16 1) -> (decimal integer string=w767:string)
        n228 = Number To Fractional String(number=w831, precision (6)=i16 2) -> (F-format string=w766:string)  [unwired: 2 in]
        n229 = Scan From String(format string="%f", input string=w837) -> (output 1=w841:dbl)  [unwired: 3 in, 3 out]
        n230 = Number To Decimal String(number=w802) -> (decimal integer string=w758:string)  [unwired: 1 in]
        n231 = Number To Fractional String(number=w799, precision (6)=i16 2) -> (F-format string=w757:string)  [unwired: 2 in]
        n232 = call "SO2 Calibration Equation.vi"("Input"=w841, "Offset"=w831, "Slope"=w830) -> ("Output"=w827:dbl)  [unwired: 12 in]
        n233 = case shown="True" w791 {
          tunnel: w829 -> [_ w995]
          tunnel: [0 w993] -> w828
          tunnel: w801 -> [_ w998]
          tunnel: w799 -> [_ w997]
          tunnel: w827 -> [_ w996]
          tunnel: [FALSE w994] -> w824
          tunnel: w790 -> [_ w992]
          frame False {
          }
          frame True {
            # "MOCCA SO2 alarm"
            n234 = case shown="True" w992 {
              tunnel: w998 -> [_ w1008]
              tunnel: w997 -> [_ w1007]
              tunnel: w996 -> [_ w1006]
              tunnel: w995 -> [w1000 w1005]
              tunnel: [w999 w1003] -> w994
              tunnel: [w1000 w1002] -> w993
              frame False {
                n235 = local read "local\ndummy"() -> (w999:bool)
              }
              frame True {
                # "check every 1 second"
                n236 = local read "MOCCA window delay time (sec)"() -> (w1004:i32)
                n237 = Select(t=w1007, s=w1008, f=w1006) -> (s? t:f=w1009:dbl)
                n238 = local read "MOCCA SO2 Limit"() -> (w1010:i32)
                n239 = To Long Integer(number=w1009) -> (32bit integer=w1011:i32)
                n240 = Greater Or Equal?(x=w1011, y=w1010) -> (x >= y?=w1001:bool)
                n241 = case shown="True" w1001 {
                  tunnel: w1005 -> [_ w1017]
                  tunnel: w1004 -> [_ w1016]
                  tunnel: [FALSE w1015] -> w1003
                  tunnel: [0 w1014] -> w1002
                  frame False {
                  }
                  frame True {
                    n242 = Increment(x=w1017) -> (x+1=w1014:i32)
                    n243 = Greater?(x=w1014, y=w1016) -> (0:w1015:bool)
                  }
                }
                "local\ndummy" <- w1003
              }
            }
          }
        }
        n244 = case shown="True" w790 {
          tunnel: w901 -> [_ w1066]
          tunnel: w827 -> [_ w1063]
          tunnel: w827 -> [_ w1065]
          tunnel: w900 -> [_ w1064]
          tunnel: w843 -> [_ w1057]
          tunnel: w842 -> [w1055 w1062]
          tunnel: w841 -> [_ w1061]
          tunnel: [w1055 w1060] -> w840
          tunnel: w839 -> [w1054 w1059]
          tunnel: [w1054 w1058] -> w838
          frame False {
          }
          frame True {
            # "SO2 monitor every second"
            n245 = local read "Mean Cal\n(default = ON)"() -> (w1056:bool)
            n246 = case shown="True" w1056 {
              tunnel: w1057 -> [_ w1077]
              tunnel: w1062 -> [w1068 w1076]
              tunnel: w1061 -> [_ w1074]
              tunnel: [w1068 w1072] -> w1060
              tunnel: w1059 -> [w1067 w1071]
              tunnel: [w1067 w1070] -> w1058
              frame False {
              }
              frame True {
                w1069 = 5 ("y")
                # "Mean offset calculation - 5 secs after ev8 is turned ON"
                n247 = Equal?(x=w1077, y=TRUE) -> (x = y?=w1079:bool)
                n248 = Increment(x=w1076) -> (x+1=w1078:i32)
                n249 = Select(t=w1078, s=w1079, f=0) -> (s? t:f=w1072:i32)
                n250 = Greater?(x=w1072, y=w1069) -> (0:w1075:bool)
                n251 = case shown="True" w1075 {
                  tunnel: w1074 -> [_ w1086]
                  tunnel: [w1081 w1085] -> w1070
                  tunnel: w1071 -> [w1081 _]
                  tunnel: w1069 -> [_ w1084]
                  frame False {
                  }
                  frame True {
                    n252 = local read "ev8 user set time"() -> (w1082:i32)
                    n253 = Subtract(x=w1082, y=w1084) -> (x-y=w1083:i32)
                    n254 = call <vilib>:"Mean PtByPt.vi"("x"=w1086, "sample length"=w1083) -> ("mean"=w1085:dbl)  [unwired: 2 in, 1 out]
                  }
                }
                "Mean Cal Offset" <- w1070
              }
            }
            n255 = Lossy Enqueue Element(queue=w1066, element=w1063) -> ()  [unwired: 1 in, 4 out]
            n256 = Lossy Enqueue Element(queue=w1064, element=w1065) -> ()  [unwired: 1 in, 4 out]
          }
        }
        n257 = Boolean To (0,1)(Boolean=w824) -> (0, 1=w826:i16)
        n258 = To Unsigned Long Integer(number=w826) -> (unsigned 32bit integer=w825:u32)
        n259 = Number To Decimal String(number=w825, width (-)=i16 1) -> (decimal integer string=w755:string)
        n260 = case shown="True" "Clear Display\nErrors" {
          frame False {
          }
          frame True {
            w1087 = errorcluster {"status"=FALSE, "code"=0, "source"=""} ("UDP Error Out")
            n261 = local write "SEPTIC TCP Error Out"(w1087) -> ()
            n262 = local write "Serial Visa Error"(w1087) -> ()
            n263 = local write "FISH TCP Error Out"(w1087) -> ()
            n264 = local write "UDP_Out_Error"(w1087) -> ()
          }
        }
        n265 = Number To Fractional String(number=w827, precision (6)=i16 5) -> (F-format string=w883:string)  [unwired: 2 in]
        n266 = Replace Array Subset(array=w745, new element=w883, index=0) -> (w882:string[])
        "Data Array UDP" <- w882
        n267 = Array To Spreadsheet String(delimiter (Tab)=",", array=w882, 3:"%s" ("format string")) -> (spreadsheet string=w935:string)
        n268 = call <vilib>:"Trim Whitespace.vi"("string"=w935, "location (both)"=w936) -> ("trimmed string"=w786:string)
        "Data String" <- w786
        n269 = Concatenate Strings(w908, w798, w789, w798, w781, w798, w787, w798, w846, w798, w845, w798, w786, w798, w785, w798, w784, w798, w783, w798, w782, w798, w780, w798, w779, w798, w778, w798, w777, w798, w776, w798, w775, w798, w774, w798, w773, w798, w772, w798, w771, w798, w770, w798, w769, w798, w768, w798, w837, w798, w767, w798, w766, w798, w765, w798, w764, w798, w763, w798, w762, w798, w761, w798, w760, w798, w759, w798, w758, w798, w757, w798, w755) -> (w751:string)
        n270 = Concatenate Strings(w789, w756, "dummy", w756, w787, w756, w781, w756, w785, w756, w784, w756, w783, w756, w782, w756, w780, w756, w779, w756, w778, w756, w777, w756, w776, w756, w775, w756, w774, w756, w773, w756, w772, w756, w771, w756, w770, w756, w769, w756, w768, w756, w767, w756, w766, w756, w765, w756, w764, w756, w763, w756, w762, w756, w761, w756, w760, w756, w759, w756, w758, w756, w757, w756, w755) -> (w754:string)
        n271 = local read "Stop File Write"() -> (w868:bool)
        n272 = call "SO2 TCP Packet_v3.1.vi"("ID"=w748, "Version"=w749, "TCP Packet In"=w754, "utc_time"=w753, "Data Array"=w745) -> ("TCP Binary Packet"=w910:string)  [unwired: 10 in]
        "TCP Binary Packet" <- w910
        n273 = Enqueue Element(queue=w912, element=w910, error in (no error)=w911) -> ()  [unwired: 1 in, 3 out]
        n274 = Enqueue Element(queue=w924, element=w910, error in (no error)=w923) -> ()  [unwired: 1 in, 3 out]
        n275 = String Length(string=w751) -> (length=w942:i32)
        n276 = Number To Decimal String(number=w942, width (-)=i16 3) -> (decimal integer string=w747:string)
        n277 = Concatenate Strings(w748, "01", w750, w747, w750, w751) -> (w744:string)
        "UDP_ASCII_Out" <- w744
        n278 = case shown="True" w790 {
          tunnel: w922 -> [_ w1090]
          tunnel: w921 -> [_ w1089]
          tunnel: w744 -> [_ w1088]
          frame False {
          }
          frame True {
            # "Send UDP data once\na second"
            n279 = Enqueue Element(queue=w1090, element=w1088, error in (no error)=w1089) -> ()  [unwired: 1 in, 3 out]
          }
        }
        n280 = local read "stop"() -> (w945:bool)
        n281 = Concatenate Strings(w748, w749, w750, w747, w750, w751) -> (w746:string)
        "ASCII_file_out" <- w746
        n282 = case shown="False" w868 {
          tunnel: w746 -> [w1049 _]
          tunnel: w875 -> [w1051 w1053]
          tunnel: w874 -> [w1050 w1052]
          tunnel: [w1046 _] -> w870
          tunnel: [w1045 _] -> w869
          frame False {
            n283 = Concatenate Strings(w1049, "\r") -> (w1047:string)
            n284 = Write to Text File(file (use dialog)=w1051, text=w1047, error in=w1050) -> (refnum out=w1046:refnum<file>, error out=w1045:errorcluster)  [unwired: 2 out]
          }
          frame True {
            n285 = Close File(refnum=w1053, error in=w1052) -> ()  [unwired: 2 out]
          }
        }
        n286 = node-c288() -> ()  [unwired: 1 in, 1 out]
      }
      n287 = node-c288() -> (w84:T4)  [unwired: 4 in]
      n288 = node-c288() -> (w86:T4)  [unwired: 4 in]
      n289 = timed-loop {
        tunnel: w90 -> [w428]
        timing: w84 -> [_]
        timing-out: [_] -> w83
        stop <- w429 stop-if-true
        # "10 minutes SO2 Average calculated every second"
        n290 = node-c288() -> ()  [unwired: 1 in, 1 out]
        n291 = Get Queue Status(queue=w428, return elements? (F)=TRUE) -> (elements=w419:dbl[])  [unwired: 1 in, 7 out]
        n292 = for {
          tunnel: w419 -> [w432] mode=indexing
          tunnel: [w436] -> w425
          shift-right: [w435] -> w423
          shift-left: i64 0 -> [w434]
          i -> [w436]
          n293 = To Quad Integer(1:w432) -> (0:w433:i64)
          n294 = Add(x=w434, y=w433) -> (x+y=w435:i64)
        }
        n295 = Increment(x=w425) -> (x+1=w420:i32)
        "q_size" <- w420
        n296 = To Double Precision Float(number=w423) -> (double precision float=w421:dbl)
        n297 = To Double Precision Float(number=w420) -> (double precision float=w422:dbl)
        n298 = Divide(x=w421, y=w422) -> (x/y=→"10min_so2_avg":dbl)
        n299 = local read "stop"() -> (w429:bool)
        n300 = node-c288() -> ()  [unwired: 1 in, 1 out]
      }
      n301 = timed-loop {
        tunnel: w89 -> [w448]
        timing: w86 -> [_]
        timing-out: [_] -> w85
        stop <- w449 stop-if-true
        # "8 hours SO2 Average calculated every second"
        n302 = node-c288() -> ()  [unwired: 1 in, 1 out]
        n303 = Get Queue Status(queue=w448, return elements? (F)=TRUE) -> (elements=w445:dbl[])  [unwired: 1 in, 7 out]
        n304 = for {
          tunnel: w445 -> [w452] mode=indexing
          tunnel: [w456] -> w444
          shift-right: [w455] -> w442
          shift-left: i64 0 -> [w454]
          i -> [w456]
          n305 = To Quad Integer(1:w452) -> (0:w453:i64)
          n306 = Add(x=w454, y=w453) -> (x+y=w455:i64)
        }
        n307 = Increment(x=w444) -> (x+1=w439:i32)
        "q_size 2" <- w439
        n308 = To Double Precision Float(number=w442) -> (double precision float=w440:dbl)
        n309 = To Double Precision Float(number=w439) -> (double precision float=w441:dbl)
        n310 = Divide(x=w440, y=w441) -> (x/y=→"8hr_so2_avg 2":dbl)
        n311 = local read "stop"() -> (w449:bool)
        n312 = node-c288() -> ()  [unwired: 1 in, 1 out]
      }
      n313 = while {
        tunnel: [w603] -> w112
        tunnel: w82 -> [w616]
        tunnel: w81 -> [w615]
        tunnel: [w614] -> w111
        tunnel: w108 -> [w613]
        shift-right: [w611] -> _
        shift-left: 0 -> [w612]
        shift-right: [w609] -> _
        shift-left: u32 0 -> [w610]
        tunnel: w93 -> [w601]
        stop <- "stop" stop-if-true
        w604 = 2
        w606 = string[] ["pmt voltage", "lamp voltage", "lamp int", "internal temp", "react temp", "pres", "flow", "flags"]
        # ">>Monitor command enter as a pair>>"
        # ">>Main commands>>"
        # ">>Monitor Command>>"
        n314 = Array Size(array=w606) -> (size(s)=w607:i32)
        n315 = Divide(x=w607, y=w604) -> (x/y=w605:dbl)
        n316 = for {
          N: w605 -> [_]
          tunnel: w616 -> [w626]
          tunnel: w615 -> [w625]
          tunnel: [w635] -> w603
          shift-right: [w633] -> w611
          shift-left: w612 -> [w634]
          shift-right: [w631] -> w609
          shift-left: w610 -> [w632]
          tunnel: [w630] -> w614
          tunnel: w613 -> [w629]
          tunnel: w606 -> [w622]
          tunnel: "so2" -> [w627]
          tunnel: w604 -> [w623]
          tunnel: w601 -> [w617]
          i -> [w624]
          # "FOR Loop runs according\nto the number of monitor commands"
          # "Assemble command:\nso2\npmt voltage\nlamp voltage\n\netc\netc\n\nso2\nflow\nflags"
          n317 = Multiply(x=w623, y=w624) -> (x*y=w620:i32)
          n318 = Array Subset(array=w622, index=w620, length=w623) -> (w621:string[])
          n319 = Build Array (concatenate)(w627, w621) -> (w628:string[])
          "Data In Array" <- w628
          n320 = node-c288() -> (w619:T4)  [unwired: 4 in]
          n321 = timed-sequence {
            timing: w619 -> [_]
            timing-out: [_] -> w618
            tunnel: w634 -> [w657]
            tunnel: w628 -> [w656]
            tunnel: w626 -> [w655]
            tunnel: w625 -> [w654]
            tunnel: w620 -> [w653]
            tunnel: w629 -> [w648]
            tunnel: [w644] -> w635
            tunnel: [w642] -> w633
            tunnel: w632 -> [w640]
            tunnel: [w639] -> w631
            tunnel: [w638] -> w630
            tunnel: w617 -> [w636]
            n322 = timed-flat-sequence {
              tunnel: w656 -> [w662]
              tunnel: w657 -> [w663]
              tunnel: [w660] -> w652
              tunnel: [w663] -> w651
              tunnel: [w662] -> w650
              tunnel: [w661] -> w649
              tunnel: w655 -> [w660]
              tunnel: [w659] -> w647
              tunnel: w654 -> [w659]
              tunnel: [w658] -> w646
              tunnel: w653 -> [w658]
              tunnel: [w676] -> w645
              tunnel: [w673] -> w643
              tunnel: w652 -> [w668]
              tunnel: w651 -> [w675]
              tunnel: w650 -> [w674]
              tunnel: [w672] -> w641
              tunnel: w649 -> [w672]
              tunnel: [w671] -> w637
              tunnel: w648 -> [w670]
              tunnel: w647 -> [w669]
              tunnel: w646 -> [w667]
              tunnel: w636 -> [w666]
              tunnel: [w738] -> w642
              tunnel: [w739] -> w644
              tunnel: w645 -> [w739]
              tunnel: w643 -> [w738]
              tunnel: w641 -> [w734]
              tunnel: w640 -> [w733]
              tunnel: [w732] -> w639
              tunnel: [w731] -> w638
              tunnel: w637 -> [w731]
              frame #0 {
                n323 = node-c288() -> ()  [unwired: 1 in, 1 out]
                n324 = node-c288() -> ()  [unwired: 1 in, 1 out]
                n325 = Tick Count (ms)() -> (millisecond timer value=w661:u32)
              }
              frame #1 {
                n326 = node-c288() -> ()  [unwired: 1 in, 1 out]
                n327 = while {
                  tunnel: [w690] -> w676
                  tunnel: w674 -> [w688]
                  tunnel: [w686] -> w671
                  tunnel: w670 -> [w685]
                  tunnel: w669 -> [w684]
                  tunnel: w668 -> [w683]
                  tunnel: w667 -> [w682]
                  shift-right: [w687] -> w673
                  shift-left: w675 -> [w689]
                  tunnel: w666 -> [w679]
                  stop <- TRUE stop-if-true
                  # "Receive data is organised as:\nDate Time so2 DATA -1\nDate Time pmt voltage DATA 0\nDate Time lamp voltage DATA 1\nDate Time so2 DATA -1\nDate Time lamp int DATA 2\nDate Time internal temp DATA 3\nDate Time so2 DATA -1\nDate Time react temp DATA 4\nDate Time pres DATA 5\nDate Time so2 DATA -1\nDate Time flow DATA 6\nDate Time flags DATA 7\n\nDate Time Read Error -2"
                  n328 = for {
                    tunnel: w684 -> [w707]
                    tunnel: [w708] -> w690
                    tunnel: w688 -> [w705] mode=indexing
                    tunnel: [w709] -> w686
                    tunnel: w685 -> [w715]
                    tunnel: w683 -> [w710]
                    tunnel: w682 -> [w704]
                    shift-right: [w719] -> w687
                    shift-left: w689 -> [w720]
                    tunnel: w679 -> [w693]
                    i -> [w697]
                    # "Acquire every 330msec for 3 times\nto make 1 second"
                    # "SO2 Acquisition Loop"
                    n329 = call "Wait"("Count(mSec)"=w693) -> ()  [unwired: 1 out]
                    n330 = Concatenate Strings("ID", w705, "\r") -> (w703:string)
                    "Command In" <- w703
                    n331 = call "SO2 Serial Packet Write.vi"("VISA resource name In"=w710, "Data in"=w703, "error in (no error)"=w707) -> ("VISA resource name Out"=w712:refnum<visa-resource-name>, "error out"=w711:errorcluster)  [unwired: 11 in]
                    n332 = call "SO2 Serial Packet Read.vi"("VISA resource In"=w712, "error in"=w711) -> ("VISA resource Out"=w709:refnum<visa-resource-name>, "Data Out"=w700:string, "error out"=w708:errorcluster)  [unwired: 11 in]
                    "RAW DATA" <- w700
                    n333 = Equal?(x=w700, y="Read Error") -> (x = y?=w698:bool)
                    n334 = Get Date/Time In Seconds() -> (seconds since 1Jan1904=w692:timestamp)
                    n335 = case shown="False" w698 {
                      tunnel: [w723 "-2"] -> w713
                      tunnel: w697 -> [w722 _]
                      tunnel: w704 -> [w721 _]
                      frame False {
                        n336 = case shown="0" w722 {
                          tunnel: ["-1" w727 w729] -> w723
                          tunnel: w721 -> [_ w725 w728]
                          frame 0 {
                            # "Make internal flag\n-1 represent so2 data"
                          }
                          frame 2 {
                            # "Make internal flag"
                            n337 = Increment(x=w725) -> (x+1=w726:i32)
                            n338 = Number To Decimal String(number=w726) -> (decimal integer string=w727:string)  [unwired: 1 in]
                          }
                          frame 1, Default {
                            # "Make internal flag"
                            n339 = Number To Decimal String(number=w728) -> (decimal integer string=w729:string)  [unwired: 1 in]
                          }
                        }
                      }
                      frame True {
                      }
                    }
                    n340 = Increment(x=w720) -> (x+1=w716:i32)
                    n341 = Unbundle(w708) -> ("status"=w717:bool)  [unwired: 2 out]
                    n342 = call <vilib>:"Trim Whitespace.vi"("string"=w700) -> ("trimmed string"=w714:string)  [unwired: 1 in]
                    n343 = To Unsigned Long Integer(number=w692) -> (unsigned 32bit integer=w696:u32)
                    n344 = Subtract(x=w696, y=u32 2082844800) -> (x-y=w691:u32)
                    n345 = Select(t=w716, s=w717, f=w720) -> (s? t:f=w719:i32)
                    n346 = call <vilib>:"Space Constant.vi"() -> ("String"=w701:string)
                    n347 = Number To Decimal String(number=w691) -> (decimal integer string=w694:string)  [unwired: 1 in]
                    n348 = Build Array(w694, w701, w714, w701, w713) -> (w702:string[])
                    n349 = Enqueue Element(queue=w715, element=w702) -> ()  [unwired: 2 in, 3 out]
                  }
                  "Number of Send & Read Error\nfrom Acquire Loop" <- w687
                  n350 = call "Wait Until Next Multiple"("Count(mSec)"=u32 1000) -> ()  [unwired: 1 out]
                }
                n351 = node-c288() -> ()  [unwired: 1 in, 1 out]
              }
              frame #2 {
                n352 = node-c288() -> ()  [unwired: 1 in, 1 out]
                n353 = Tick Count (ms)() -> (millisecond timer value=w737:u32)
                n354 = Subtract(x=w737, y=w734) -> (x-y=w736:u32)
                "Acq Time" <- w736
                "Time taken history" <- w736
                n355 = Greater?(x=w736, y=w733) -> (0:w735:bool)
                n356 = Select(t=w736, s=w735, f=w733) -> (s? t:f=w732:u32)
                "Max Acq Time diff" <- w732
                n357 = node-c288() -> ()  [unwired: 1 in, 1 out]
              }
            }
          }
          n358 = node-c288(w618) -> ()  [unwired: 1 out]
        }
      }
      n359 = node-c288(w85) -> ()  [unwired: 1 out]
      n360 = node-c288(w83) -> ()  [unwired: 1 out]
      n361 = while {
        stop <- FALSE stop-if-true
        # "CAL MFC 3 status & control"
        n362 = Wait (ms)(milliseconds to wait=u32 1000) -> ()  [unwired: 1 out]
        n363 = call-poly "VISA Configure Serial Port"("VISA resource name"="VISA resource name 2", "timeout (10sec)"="timeout (10sec) 2", "termination char\n(0xA = '\\n' = LF)"=u8 13 ("termination char\n(0xA = '\\n' = LF)"), "Enable Termination\nChar (T)"=TRUE ("Enable Termination\nChar (T)"), "baud rate (9600)"=u32 19200) -> ("VISA resource name out"=w360:refnum<visa-resource-name>, "error out"=w356:errorcluster)  [unwired: 9 in]
        n364 = case shown="No Error" w356 {
          selector: w356 -> [w367 w417]
          tunnel: w360 -> [w368 w418]
          tunnel: [w366 w418] -> w359
          tunnel: [w365 w417] -> w358
          frame No Error {
            n365 = node-c288() -> (w363:T4)  [unwired: 4 in]
            n366 = timed-loop {
              tunnel: w368 -> [w391]
              tunnel: w367 -> [w389]
              tunnel: [w382] -> w366
              tunnel: [w377] -> w365
              shift-right: [w378] -> _
              shift-left: FALSE -> [w381]
              timing: w363 -> [_]
              timing-out: [_] -> w362
              shift-right: [w369] -> _
              shift-left: 0.0 -> [w371]
              stop <- w377 stop-if-true
              n367 = node-c288() -> ()  [unwired: 1 in, 1 out]
              n368 = local read "MFC_3 SLPM set value"() -> (w369:dbl)
              n369 = Not Equal?(x=w369, y=w371) -> (x != y?=w370:bool)
              n370 = case shown="True" w370 {
                tunnel: w391 -> [w399 w414]
                tunnel: [w399 w414] -> w390
                tunnel: w389 -> [w398 w413]
                tunnel: [w398 w413] -> w388
                tunnel: "A" -> [w402 w406]
                tunnel: [w400 w403] -> w386
                frame False {
                  n371 = Concatenate Strings(w402, "\r") -> (w400:string)
                }
                frame True {
                  n372 = Multiply(x="MFC_3 SLPM set value", y=u32 64000) -> (x*y=w410:dbl)
                  n373 = Divide(x=w410, y=u32 5) -> (x/y=w408:dbl)
                  n374 = To Unsigned Long Integer(number=w408) -> (unsigned 32bit integer=w407:u32)
                  n375 = Number To Decimal String(number=w407) -> (decimal integer string=w405:string)  [unwired: 1 in]
                  n376 = Concatenate Strings(w406, w405, "\r") -> (w403:string)
                }
              }
              n377 = VISA Flush I/O Buffer(VISA resource name=w390, error in (no error)=w388) -> (VISA resource name out=w393:refnum<visa-resource-name>, error out=w392:errorcluster)  [unwired: 1 in]
              n378 = Select(t=FALSE, s=w381, f=TRUE) -> (s? t:f=w378:bool)
              "status" <- w378
              n379 = VISA Write(VISA resource name=w393, write buffer=w386, error in (no error)=w392) -> (VISA resource name out=w385:refnum<visa-resource-name>, error out=w384:errorcluster)  [unwired: 1 out]
              n380 = VISA Flush I/O Buffer(VISA resource name=w385, error in (no error)=w384) -> (VISA resource name out=w395:refnum<visa-resource-name>, error out=w394:errorcluster)  [unwired: 1 in]
              n381 = VISA Read(VISA resource name=w395, byte count=u32 50, error in (no error)=w394) -> (VISA resource name out=w382:refnum<visa-resource-name>, read buffer=w376:string, error out=w377:errorcluster)  [unwired: 1 out]
              "Value Read 3" <- w376
              n382 = call <vilib>:"Space Constant.vi"() -> ("String"=w375:string)
              n383 = Spreadsheet String To Array(delimiter (Tab)=w375, format string="%f", spreadsheet string=w376, array type (2D Dbl)=dbl[] []) -> (array=→"MFC 3":dbl[])
              n384 = node-c288() -> ()  [unwired: 1 in, 1 out]
            }
            n385 = node-c288(w362) -> ()  [unwired: 1 out]
          }
          frame Error {
          }
        }
        n386 = VISA Close(VISA resource name=w359, error in (no error)=w358) -> (error out=→"error out 3":errorcluster)
      }
      n387 = while {
        stop <- FALSE stop-if-true
        # "CAL MFC 2 status & control"
        n388 = Wait (ms)(milliseconds to wait=u32 1000) -> ()  [unwired: 1 out]
        n389 = call-poly "VISA Configure Serial Port"("VISA resource name"="VISA resource name 3", "timeout (10sec)"="timeout (10sec) 3", "termination char\n(0xA = '\\n' = LF)"=u8 13 ("termination char\n(0xA = '\\n' = LF)"), "Enable Termination\nChar (T)"=TRUE ("Enable Termination\nChar (T)"), "baud rate (9600)"=u32 19200) -> ("VISA resource name out"=w290:refnum<visa-resource-name>, "error out"=w286:errorcluster)  [unwired: 9 in]
        n390 = case shown="No Error" w286 {
          selector: w286 -> [w297 w347]
          tunnel: w290 -> [w298 w348]
          tunnel: [w296 w348] -> w289
          tunnel: [w295 w347] -> w288
          frame No Error {
            n391 = node-c288() -> (w293:T4)  [unwired: 4 in]
            n392 = timed-loop {
              tunnel: w298 -> [w321]
              tunnel: w297 -> [w319]
              tunnel: [w312] -> w296
              tunnel: [w307] -> w295
              shift-right: [w308] -> _
              shift-left: FALSE -> [w311]
              timing: w293 -> [_]
              timing-out: [_] -> w292
              shift-right: [w299] -> _
              shift-left: 0.0 -> [w301]
              stop <- w307 stop-if-true
              n393 = node-c288() -> ()  [unwired: 1 in, 1 out]
              n394 = local read "MFC_2 SLPM set value"() -> (w299:dbl)
              n395 = Not Equal?(x=w299, y=w301) -> (x != y?=w300:bool)
              n396 = case shown="True" w300 {
                tunnel: w321 -> [w329 w344]
                tunnel: [w329 w344] -> w320
                tunnel: w319 -> [w328 w343]
                tunnel: [w328 w343] -> w318
                tunnel: "A" -> [w332 w336]
                tunnel: [w330 w333] -> w316
                frame False {
                  n397 = Concatenate Strings(w332, "\r") -> (w330:string)
                }
                frame True {
                  n398 = Multiply(x="MFC_2 SLPM set value", y=u32 64000) -> (x*y=w340:dbl)
                  n399 = Divide(x=w340, y=u32 5) -> (x/y=w338:dbl)
                  n400 = To Unsigned Long Integer(number=w338) -> (unsigned 32bit integer=w337:u32)
                  n401 = Number To Decimal String(number=w337) -> (decimal integer string=w335:string)  [unwired: 1 in]
                  n402 = Concatenate Strings(w336, w335, "\r") -> (w333:string)
                }
              }
              n403 = Select(t=FALSE, s=w311, f=TRUE) -> (s? t:f=w308:bool)
              "status 2" <- w308
              n404 = VISA Flush I/O Buffer(VISA resource name=w320, error in (no error)=w318) -> (VISA resource name out=w323:refnum<visa-resource-name>, error out=w322:errorcluster)  [unwired: 1 in]
              n405 = VISA Write(VISA resource name=w323, write buffer=w316, error in (no error)=w322) -> (VISA resource name out=w315:refnum<visa-resource-name>, error out=w314:errorcluster)  [unwired: 1 out]
              n406 = VISA Flush I/O Buffer(VISA resource name=w315, error in (no error)=w314) -> (VISA resource name out=w325:refnum<visa-resource-name>, error out=w324:errorcluster)  [unwired: 1 in]
              n407 = VISA Read(VISA resource name=w325, byte count=u32 50, error in (no error)=w324) -> (VISA resource name out=w312:refnum<visa-resource-name>, read buffer=w306:string, error out=w307:errorcluster)  [unwired: 1 out]
              "Value Read 2" <- w306
              n408 = call <vilib>:"Space Constant.vi"() -> ("String"=w305:string)
              n409 = Spreadsheet String To Array(delimiter (Tab)=w305, format string="%f", spreadsheet string=w306, array type (2D Dbl)=dbl[] []) -> (array=→"MFC 2":dbl[])
              n410 = node-c288() -> ()  [unwired: 1 in, 1 out]
            }
            n411 = node-c288(w292) -> ()  [unwired: 1 out]
          }
          frame Error {
          }
        }
        n412 = VISA Close(VISA resource name=w289, error in (no error)=w288) -> (error out=→"error out 2":errorcluster)
      }
      n413 = node-c288(w109) -> ()  [unwired: 1 out]
      n414 = while {
        stop <- FALSE stop-if-true
        n415 = node-c288() -> (w119:T4)  [unwired: 4 in]
        n416 = Create Network Stream Reader Endpoint(7:10 ("reader buffer size"), 9:T3 {"Message"="", "Message Data"=variant} ("Message Cluster"), 11:"/command/reader/SO2" ("reader url")) -> (0:w125:errorcluster, 3:w126:refnum<k21>)  [unwired: 4 in]
        n417 = timed-loop "Host->Target Command Reader" {
          shift-right: [w136] -> w123
          shift-left: w125 -> [w139]
          shift-right: [w137] -> w122
          shift-left: w126 -> [w138]
          tunnel: [TRUE] -> _
          timing: w119 -> [_]
          timing-out: [_] -> w118
          stop <- w130 stop-if-true
          # "Receive Commands from Host VI"
          n418 = node-c288() -> ()  [unwired: 1 in, 1 out]
          n419 = shared-variable-read(w138, w139) -> (w137:refnum<k21>, w132:errorcluster, w134:bool, w135:T3)  [unwired: 1 in]
          n420 = Or(x=w134, y=w132) -> (x .or. y?=w133:bool)
          n421 = case shown="False" w133 {
            selector: w133 -> [_ w275]
            tunnel: w132 -> [w147 w276]
            tunnel: [w146 w276] -> w136
            tunnel: w135 -> [w144 _]
            tunnel: [w145 w275] -> w130
            frame False {
              n422 = Unbundle By Name(w144) -> ("Message"=w143:string, "Message Data"=w142:variant)
              n423 = case shown="\"V6\"" w143 {
                tunnel: w147 -> [w149 w154 w159 w164 w169 w174 w179 w184 w189 w194 w199 w204 w209 w214 w219 w224 w229 w234 w239 w244 w249 w254 w259 w263 w268 w273]
                tunnel: [w149 w153 w158 w163 w168 w173 w178 w183 w188 w193 w198 w203 w208 w213 w218 w223 w228 w233 w238 w243 w248 w253 w258 w261 w266 w271] -> w146
                tunnel: w142 -> [_ w152 w157 w162 w167 w172 w177 w182 w187 w192 w197 w202 w207 w212 w217 w222 w227 w232 w237 w242 w247 w252 w257 w264 w269 w274]
                tunnel: [TRUE _ _ _ _ _ _ _ _ _ _ _ _ _ _ _ _ _ _ _ _ _ _ _ _ _] -> w145
                frame "Stop", Default {
                }
                frame "V9" {
                  n424 = Variant To Data(error in=w154, type=FALSE, Variant=w152) -> (data=w150:bool, error out=w153:errorcluster)
                  "V9" <- w150
                  n425 = shared-variable "NI-cRIO9022-019C2C95\\Mod6\\DO7"(w150) -> ()  [unwired: 1 in, 1 out]
                }
                frame "MFC_2" {
                  n426 = Variant To Data(error in=w159, type=0.0, Variant=w157) -> (data=w155:dbl, error out=w158:errorcluster)
                  n427 = local write "MFC_2 SLPM set value"(w155) -> ()
                }
                frame "cal_gas_cylin_conc" {
                  n428 = Variant To Data(error in=w164, type=0.0, Variant=w162) -> (data=→"cal gas cylinder conc":dbl, error out=w163:errorcluster)
                }
                frame "sim_MOCCA_conc" {
                  n429 = Variant To Data(error in=w169, type=0.0, Variant=w167) -> (data=→"Simulate MOCCA Conc":dbl, error out=w168:errorcluster)
                }
                frame "Auto_zero" {
                  n430 = Variant To Data(error in=w174, type=FALSE, Variant=w172) -> (data=→"Auto Zeroing":bool, error out=w173:errorcluster)
                }
                frame "zeroing_interval" {
                  n431 = Variant To Data(error in=w179, type=0, Variant=w177) -> (data=→"ev8 zero interval":i32, error out=w178:errorcluster)
                }
                frame "MOCCA_window_delay_time" {
                  n432 = Variant To Data(error in=w184, type=0, Variant=w182) -> (data=→"MOCCA window delay time (sec)":i32, error out=w183:errorcluster)
                }
                frame "MOCCA_limit" {
                  n433 = Variant To Data(error in=w189, type=0, Variant=w187) -> (data=→"MOCCA SO2 Limit":i32, error out=w188:errorcluster)
                }
                frame "eV8_user_set_time" {
                  n434 = Variant To Data(error in=w194, type=0, Variant=w192) -> (data=→"ev8 user set time":i32, error out=w193:errorcluster)
                }
                frame "MFC_3" {
                  n435 = Variant To Data(error in=w199, type=0.0, Variant=w197) -> (data=w195:dbl, error out=w198:errorcluster)
                  n436 = local write "MFC_3 SLPM set value"(w195) -> ()
                }
                frame "Simulate STEL Conc" {
                  n437 = Variant To Data(error in=w204, type=0.0, Variant=w202) -> (data=→"Simulate STEL Conc":dbl, error out=w203:errorcluster)
                }
                frame "Simulate TWA Conc" {
                  n438 = Variant To Data(error in=w209, type=0.0, Variant=w207) -> (data=→"Simulate TWA Conc":dbl, error out=w208:errorcluster)
                }
                frame "Offset" {
                  n439 = Variant To Data(error in=w214, type=0.0, Variant=w212) -> (data=→"Zero":dbl, error out=w213:errorcluster)
                }
                frame "10mins STEL Limit" {
                  n440 = Variant To Data(error in=w219, type=0, Variant=w217) -> (data=→"10mins_STEL_limit":i32, error out=w218:errorcluster)
                }
                frame "UDP Time Offset" {
                  n441 = Variant To Data(error in=w224, type=0, Variant=w222) -> (data=→"UDP Time Stamp Offset":i32, error out=w223:errorcluster)
                }
                frame "8hr TWA Limit" {
                  n442 = Variant To Data(error in=w229, type=0, Variant=w227) -> (data=→"8hr_TWA_limit":i32, error out=w228:errorcluster)
                }
                frame "Slope" {
                  n443 = Variant To Data(error in=w234, type=0.0, Variant=w232) -> (data=→"Slope":dbl, error out=w233:errorcluster)
                }
                frame "V8" {
                  n444 = Variant To Data(error in=w239, type=FALSE, Variant=w237) -> (data=w235:bool, error out=w238:errorcluster)
                  "V8" <- w235
                  n445 = shared-variable "NI-cRIO9022-019C2C95\\Mod6\\DO6"(w235) -> ()  [unwired: 1 in, 1 out]
                }
                frame "Stop File Write" {
                  n446 = Variant To Data(error in=w244, type=FALSE, Variant=w242) -> (data=→"Stop File Write":bool, error out=w243:errorcluster)
                }
                frame "SO2_MOCCA_Alarm" {
                  n447 = Variant To Data(error in=w249, type=FALSE, Variant=w247) -> (data=→"SO2 Inflight MOCCA Alarm\n(default = OFF)":bool, error out=w248:errorcluster)
                }
                frame "Flight Number" {
                  n448 = Variant To Data(error in=w254, type="", Variant=w252) -> (data=→"Flight Number":string, error out=w253:errorcluster)
                }
                frame "V6" {
                  n449 = Variant To Data(error in=w259, type=FALSE, Variant=w257) -> (data=w255:bool, error out=w258:errorcluster)
                  "V6" <- w255
                  n450 = shared-variable "NI-cRIO9022-019C2C95\\Mod6\\DO4"(w255) -> ()  [unwired: 1 in, 1 out]
                }
                frame "Simulate Conc" {
                  n451 = Variant To Data(error in=w263, type=FALSE, Variant=w264) -> (data=→"Simulate\nconc":bool, error out=w261:errorcluster)
                }
                frame "calcon_save" {
                  n452 = Variant To Data(error in=w268, type=FALSE, Variant=w269) -> (data=→"calcon save to file":bool, error out=w266:errorcluster)
                }
                frame "mean_cal_status" {
                  n453 = Variant To Data(error in=w273, type=FALSE, Variant=w274) -> (data=→"Mean Cal\n(default = ON)":bool, error out=w271:errorcluster)
                }
              }
            }
            frame True {
            }
          }
          n454 = node-c288() -> ()  [unwired: 1 in, 1 out]
        }
        n455 = node-c288(w118) -> ()  [unwired: 1 out]
        n456 = Destroy Stream Endpoint(8:w123, 11:w122) -> (0:→"error out 4":errorcluster)
        n457 = Wait (ms)(milliseconds to wait=u32 1000) -> ()  [unwired: 1 out]
      }
      n458 = while {
        tunnel: w96 -> [w502]
        stop <- w503 stop-if-true
        # "UDP Broadcast loop"
        # "Broadcast UDP SO2 Data"
        n459 = node-c288() -> (w505:T4)  [unwired: 4 in]
        n460 = String To IP(1:"239.1.4.6" ("name")) -> (0:w507:u32)
        n461 = call-poly <vilib>:"UDP Multicast Open.vi"("time-to-live (1)"=u16 5, "port"=u16 10001) -> ("error out"=w515:errorcluster, "connection ID"=w516:refnum<k16>)  [unwired: 8 in]
        n462 = timed-loop {
          tunnel: w516 -> [w536]
          tunnel: w515 -> [w535]
          tunnel: [w522] -> w511
          shift-right: [w525] -> _
          shift-left: FALSE -> [w528]
          tunnel: [w520] -> w509
          tunnel: w507 -> [w524]
          tunnel: u16 50001 ("port or service name") -> [w523]
          timing: w505 -> [_]
          timing-out: [_] -> w504
          tunnel: [w518] -> w503
          tunnel: w502 -> [w517]
          stop <- w519 stop-if-true
          n463 = node-c288() -> ()  [unwired: 1 in, 1 out]
          n464 = local read "Flight Number"() -> (w531:string)
          n465 = Select(t=FALSE, s=w528, f=TRUE) -> (s? t:f=w525:bool)
          "UDP packet \nstatus" <- w525
          n466 = feedback-in #2(w531) -> ()
          n467 = feedback #2() -> (w530:string)  [unwired: 1 in]
          n468 = Not Equal?(x=w531, y=w530) -> (x != y?=w529:bool)
          n469 = flat-sequence {
            tunnel: w524 -> [w544]
            tunnel: w535 -> [w545]
            tunnel: w536 -> [w546]
            tunnel: [w546] -> w534
            tunnel: [w545] -> w533
            tunnel: [w544] -> w532
            tunnel: w529 -> [w543]
            tunnel: w523 -> [w556]
            tunnel: w534 -> [w555]
            tunnel: w533 -> [w554]
            tunnel: w532 -> [w553]
            tunnel: [w552] -> w522
            tunnel: [w551] -> w520
            tunnel: w517 -> [w550]
            frame #0 {
              n470 = feedback #3(u32 0) -> (w540:u32)
              n471 = case shown="True" w543 {
                tunnel: w540 -> [w547 _]
                tunnel: [w547 u32 0] -> w539
                frame False {
                }
                frame True {
                }
              }
              "UDP_Pack_num" <- w539
              n472 = Increment(x=w539) -> (x+1=w541:u32)
              n473 = feedback-in #3(w541) -> ()
            }
            frame #1 {
              n474 = Dequeue Element(queue=w550) -> (element=w549:string)  [unwired: 2 in, 3 out]
              n475 = UDP Write(address=w553, port or service name=w556, connection ID=w555, data in=w549, 8:w554) -> (error out=w551:errorcluster, 3:w552:refnum<k16>)  [unwired: 1 in]
            }
          }
          n476 = local read "stop"() -> (w518:bool)
          n477 = Unbundle(w520) -> ("status"=w521:bool)  [unwired: 2 out]
          n478 = node-c288() -> ()  [unwired: 1 in, 1 out]
          n479 = Compound Arithmetic op=OR(w521, w518) -> (w519:bool)
        }
        n480 = node-c288(w504) -> ()  [unwired: 1 out]
        n481 = UDP Close(connection ID=w511, 8:w509) -> (error out=→"UDP_Out_Error":errorcluster)  [unwired: 1 out]
        n482 = Wait (ms)(milliseconds to wait=u32 1000) -> ()  [unwired: 1 out]
      }
      n483 = while {
        stop <- FALSE stop-if-true
        # "Emergency shutdown on the valves when connection to the client drops"
        n484 = shared-variable ".\\Global Shared Variables.lvlib\\Disconnect_WatchDog"() -> (w113:bool)  [unwired: 1 in, 1 out]
        n485 = Wait (ms)(milliseconds to wait=u32 1000) -> ()  [unwired: 1 out]
        n486 = case shown="True" w113 {
          frame False {
          }
          frame True {
            w116 = FALSE
            n487 = shared-variable "NI-cRIO9022-019C2C95\\Mod6\\DO4"(w116) -> ()  [unwired: 1 in, 1 out]
            n488 = shared-variable "NI-cRIO9022-019C2C95\\Mod6\\DO7"(w116) -> ()  [unwired: 1 in, 1 out]
            n489 = shared-variable "NI-cRIO9022-019C2C95\\Mod6\\DO6"(w116) -> ()  [unwired: 1 in, 1 out]
            n490 = local write "MFC_2 SLPM set value"(0.0 ("MFC_2 SLPM set value")) -> ()
          }
        }
      }
      n491 = while {
        tunnel: w94 -> [w461]
        tunnel: w95 -> [w460]
        stop <- w464 stop-if-true
        # "TCP Loop writing to SEPTIC Tank"
        n492 = TCP Open Connection(address="192.168.101.108", remote port or service name=u16 3502) -> (connection ID=w467:refnum<k5>, error out=w462:errorcluster)  [unwired: 3 in]
        n493 = case shown="No Error" w462 {
          selector: w462 -> [w472 w499]
          tunnel: w467 -> [w477 w500]
          tunnel: [w476 w500] -> w466
          tunnel: [w475 w499] -> w465
          tunnel: [w474 w498] -> w464
          tunnel: w460 -> [w471 _]
          tunnel: w461 -> [w470 _]
          frame No Error {
            n494 = node-c288() -> (w479:T4)  [unwired: 4 in]
            n495 = timed-loop {
              tunnel: w477 -> [w493]
              tunnel: w472 -> [w492]
              tunnel: [w491] -> w476
              tunnel: [w490] -> w475
              tunnel: [w480] -> w474
              shift-right: [w484] -> _
              shift-left: FALSE -> [w487]
              timing: w479 -> [_]
              timing-out: [_] -> w478
              tunnel: w471 -> [w483]
              tunnel: w470 -> [w482]
              stop <- w488 stop-if-true
              n496 = node-c288() -> ()  [unwired: 1 in, 1 out]
              n497 = Dequeue Element(queue=w483, error in (no error)=w482) -> (element=w481:string)  [unwired: 1 in, 3 out]
              n498 = Select(t=FALSE, s=w487, f=TRUE) -> (s? t:f=w484:bool)
              "TCP packet\nSend to SEPTIC" <- w484
              n499 = TCP Write(connection ID=w493, data in=w481, error in (no error)=w492) -> (connection ID out=w491:refnum<k5>, error out=w490:errorcluster)  [unwired: 1 in, 1 out]
              n500 = local read "stop"() -> (w480:bool)
              n501 = Unbundle(w490) -> ("status"=w489:bool)  [unwired: 2 out]
              n502 = node-c288() -> ()  [unwired: 1 in, 1 out]
              n503 = Compound Arithmetic op=OR(w489, w480) -> (w488:bool)
            }
            n504 = node-c288(w478) -> ()  [unwired: 1 out]
          }
          frame Error {
            n505 = local read "stop"() -> (w498:bool)
          }
        }
        n506 = TCP Close Connection(connection ID=w466, error in (no error)=w465) -> (error out=→"SEPTIC TCP Error Out":errorcluster)  [unwired: 1 in, 1 out]
        n507 = Wait (ms)(milliseconds to wait=u32 1000) -> ()  [unwired: 1 out]
      }
      n508 = while {
        tunnel: w100 -> [w561]
        tunnel: w99 -> [w560]
        stop <- w564 stop-if-true
        # "TCP Loop writing to FISH Tank"
        n509 = TCP Open Connection(address="192.168.101.110", remote port or service name=u16 3502) -> (connection ID=w567:refnum<k5>, error out=w562:errorcluster)  [unwired: 3 in]
        n510 = case shown="No Error" w562 {
          selector: w562 -> [w572 w599]
          tunnel: w567 -> [w577 w600]
          tunnel: [w576 w600] -> w566
          tunnel: [w575 w599] -> w565
          tunnel: [w574 w598] -> w564
          tunnel: w561 -> [w571 _]
          tunnel: w560 -> [w570 _]
          frame No Error {
            n511 = node-c288() -> (w579:T4)  [unwired: 4 in]
            n512 = timed-loop {
              tunnel: w577 -> [w593]
              tunnel: w572 -> [w592]
              tunnel: [w591] -> w576
              tunnel: [w590] -> w575
              tunnel: [w587] -> w574
              shift-right: [w583] -> _
              shift-left: FALSE -> [w586]
              timing: w579 -> [_]
              timing-out: [_] -> w578
              tunnel: w571 -> [w582]
              tunnel: w570 -> [w581]
              stop <- w588 stop-if-true
              n513 = node-c288() -> ()  [unwired: 1 in, 1 out]
              n514 = Dequeue Element(queue=w582, error in (no error)=w581) -> (element=w580:string)  [unwired: 1 in, 3 out]
              n515 = Select(t=FALSE, s=w586, f=TRUE) -> (s? t:f=w583:bool)
              "TCP packet\nSend to FISH" <- w583
              n516 = TCP Write(connection ID=w593, data in=w580, error in (no error)=w592) -> (connection ID out=w591:refnum<k5>, error out=w590:errorcluster)  [unwired: 1 in, 1 out]
              n517 = local read "stop"() -> (w587:bool)
              n518 = Unbundle(w590) -> ("status"=w589:bool)  [unwired: 2 out]
              n519 = node-c288() -> ()  [unwired: 1 in, 1 out]
              n520 = Compound Arithmetic op=OR(w589, w587) -> (w588:bool)
            }
            n521 = node-c288(w578) -> ()  [unwired: 1 out]
          }
          frame Error {
            n522 = local read "stop"() -> (w598:bool)
          }
        }
        n523 = TCP Close Connection(connection ID=w566, error in (no error)=w565) -> (error out=→"FISH TCP Error Out":errorcluster)  [unwired: 1 in, 1 out]
        n524 = Wait (ms)(milliseconds to wait=u32 1000) -> ()  [unwired: 1 out]
      }
    }
    frame Error {
    }
  }
  n525 = VISA Close(VISA resource name=w36, error in (no error)=w35) -> (error out=→"Serial Visa Error":errorcluster)
